vi "SO2 43i Serial Data Recording & DECADEv4.1.vi"() -> ()   [LabVIEW 2014]
uses:
  <vilib>/Instr/_visa.llb/VISA Set IO Buffer Mask.ctl
  <vilib>/Platform/TimedLoop/XDataNode/timing_clust.ctl
  <vilib>/Platform/TimedLoop/XDataNode/nitl_modes.ctl
  <vilib>/Platform/TimedLoop/XDataNode/wakeup.ctl
  C:/Program Files (x86)/National Instruments/LabVIEW 2014/examples/Data Communication/Network Streams/Simple Network Streams/support/Network Stream Command.ctl
  <vilib>/Utility/error.llb/whitespace.ctl
  <vilib>/Instr/_visa.llb/VISA Configure Serial Port (Instr).vi
  <vilib>/Utility/file.llb/Read From Spreadsheet File (string).vi
  <vilib>/Utility/tcp.llb/UDP Multicast Write-Only Open.vi
  <vilib>/platform/TimedLoop/XDataNode/XDataNode.xnode
  <vilib>/Platform/TimedLoop/XDataNode/XDNodeRunTimeDep.lvlib
  <vilib>/ptbypt/NI_PtbyPt.lvlib
panel:
  out "local\ndummy":bool
  out "cal gas cylinder conc":dbl=500.0 format="%.4g"
  out "calcon save to file":bool
  out "ev8 zero interval":i32=600
  out "Auto Zeroing":bool
  out "Simulate MOCCA Conc":dbl
  out "MOCCA window delay time (sec)":i32=30
  out "MOCCA SO2 Limit":i32=800
  out "SO2 Inflight MOCCA Alarm\n(default = OFF)":bool
  out "ev8 user set time":i32=60
  out "Mean Cal Offset":dbl
  out "Mean Cal\n(default = ON)":bool=TRUE
  out "Default file name":string
  out "Stop File Write":bool
  out "error out 4":errorcluster
  out "V6":bool
  out "V8":bool
  out "V9":bool
  out "error out 2":errorcluster
  in  "MFC_2 SLPM set value":dbl
  out "Value Read 2":string
  out "status 2":bool
  out "MFC 2":dbl[](array[numeric])
  in  "VISA resource name 3":refnum<visa-resource-name>="ASRL4::INSTR"
  in  "timeout (10sec) 3":u32=3000
  out "error out 3":errorcluster
  in  "MFC_3 SLPM set value":dbl=2.0
  out "Value Read 3":string
  out "status":bool
  out "MFC 3":dbl[](array[numeric])
  in  "VISA resource name 2":refnum<visa-resource-name>="ASRL5::INSTR"
  in  "timeout (10sec) 2":u32=3000
  out "Data Array UDP":string[](array[string])
  out "Slope":dbl=1.1
  out "Zero":dbl
  out "Simulate TWA Conc":dbl
  out "8hr_TWA_limit":i32=490
  out "10mins_STEL_limit":i32=800
  out "Simulate STEL Conc":dbl
  out "Simulate\nconc":bool
  out "q_size 2":i32
  out "8hr_so2_avg 2":dbl=1.0
  out "10min_so2_avg":dbl=1.0
  out "q_size":i32
  in  "Clear Display\nErrors":bool
  out "Data Processing":bool
  out "Serial Visa Error":errorcluster
  out "SEPTIC TCP Error Out":errorcluster
  out "TCP packet\nSend to SEPTIC":bool
  out "UDP Time Stamp Offset":i32=1
  out "Data Array TCP":string[](array[string])
  out "UDP packet \nstatus":bool
  out "UDP_Out_Error":errorcluster
  out "FISH TCP Error Out":errorcluster
  out "TCP packet\nSend to FISH":bool
  out "TCP Binary Packet":string
  out "Scan from String Error Counter\nfrom process loop":i32
  out "Read Error Counter\nfrom process loop":i32
  in  "milliseconds to wait":u32=330
  in  "ID":string="µ"
  in  "VISA resource name":refnum<visa-resource-name>="ASRL6::INSTR"
  out "Data In Array":string[](array[string])
  out "UDP_ASCII_Out":string
  out "UDP_Pack_num":u32
  out "Flight Number":string
  in  "dummy":string="00"
  out "Data String":string
  out "Internal packet":string[](array[string])
  out "RAW DATA":string
  in  "stop":bool
  out "Time taken history":u32(graph)
  out "Max Acq Time diff":u32
  out "Acq Time":u32
  out "Number of Send & Read Error\nfrom Acquire Loop":i32
  out "Command In":string
  # "SO2_conc"
  # "PMT_Volt"
  # "Lamp_Volt"
  # "Lamp_Intensity_Hz"
  # "Internal_Temp_degC"
  # "Reaction_Chamber_Temp_degC"
  # "Reaction_Chamber_Press_mmHg"
  # "Sample_Flow_litre_per_minute"
  # "Flag"
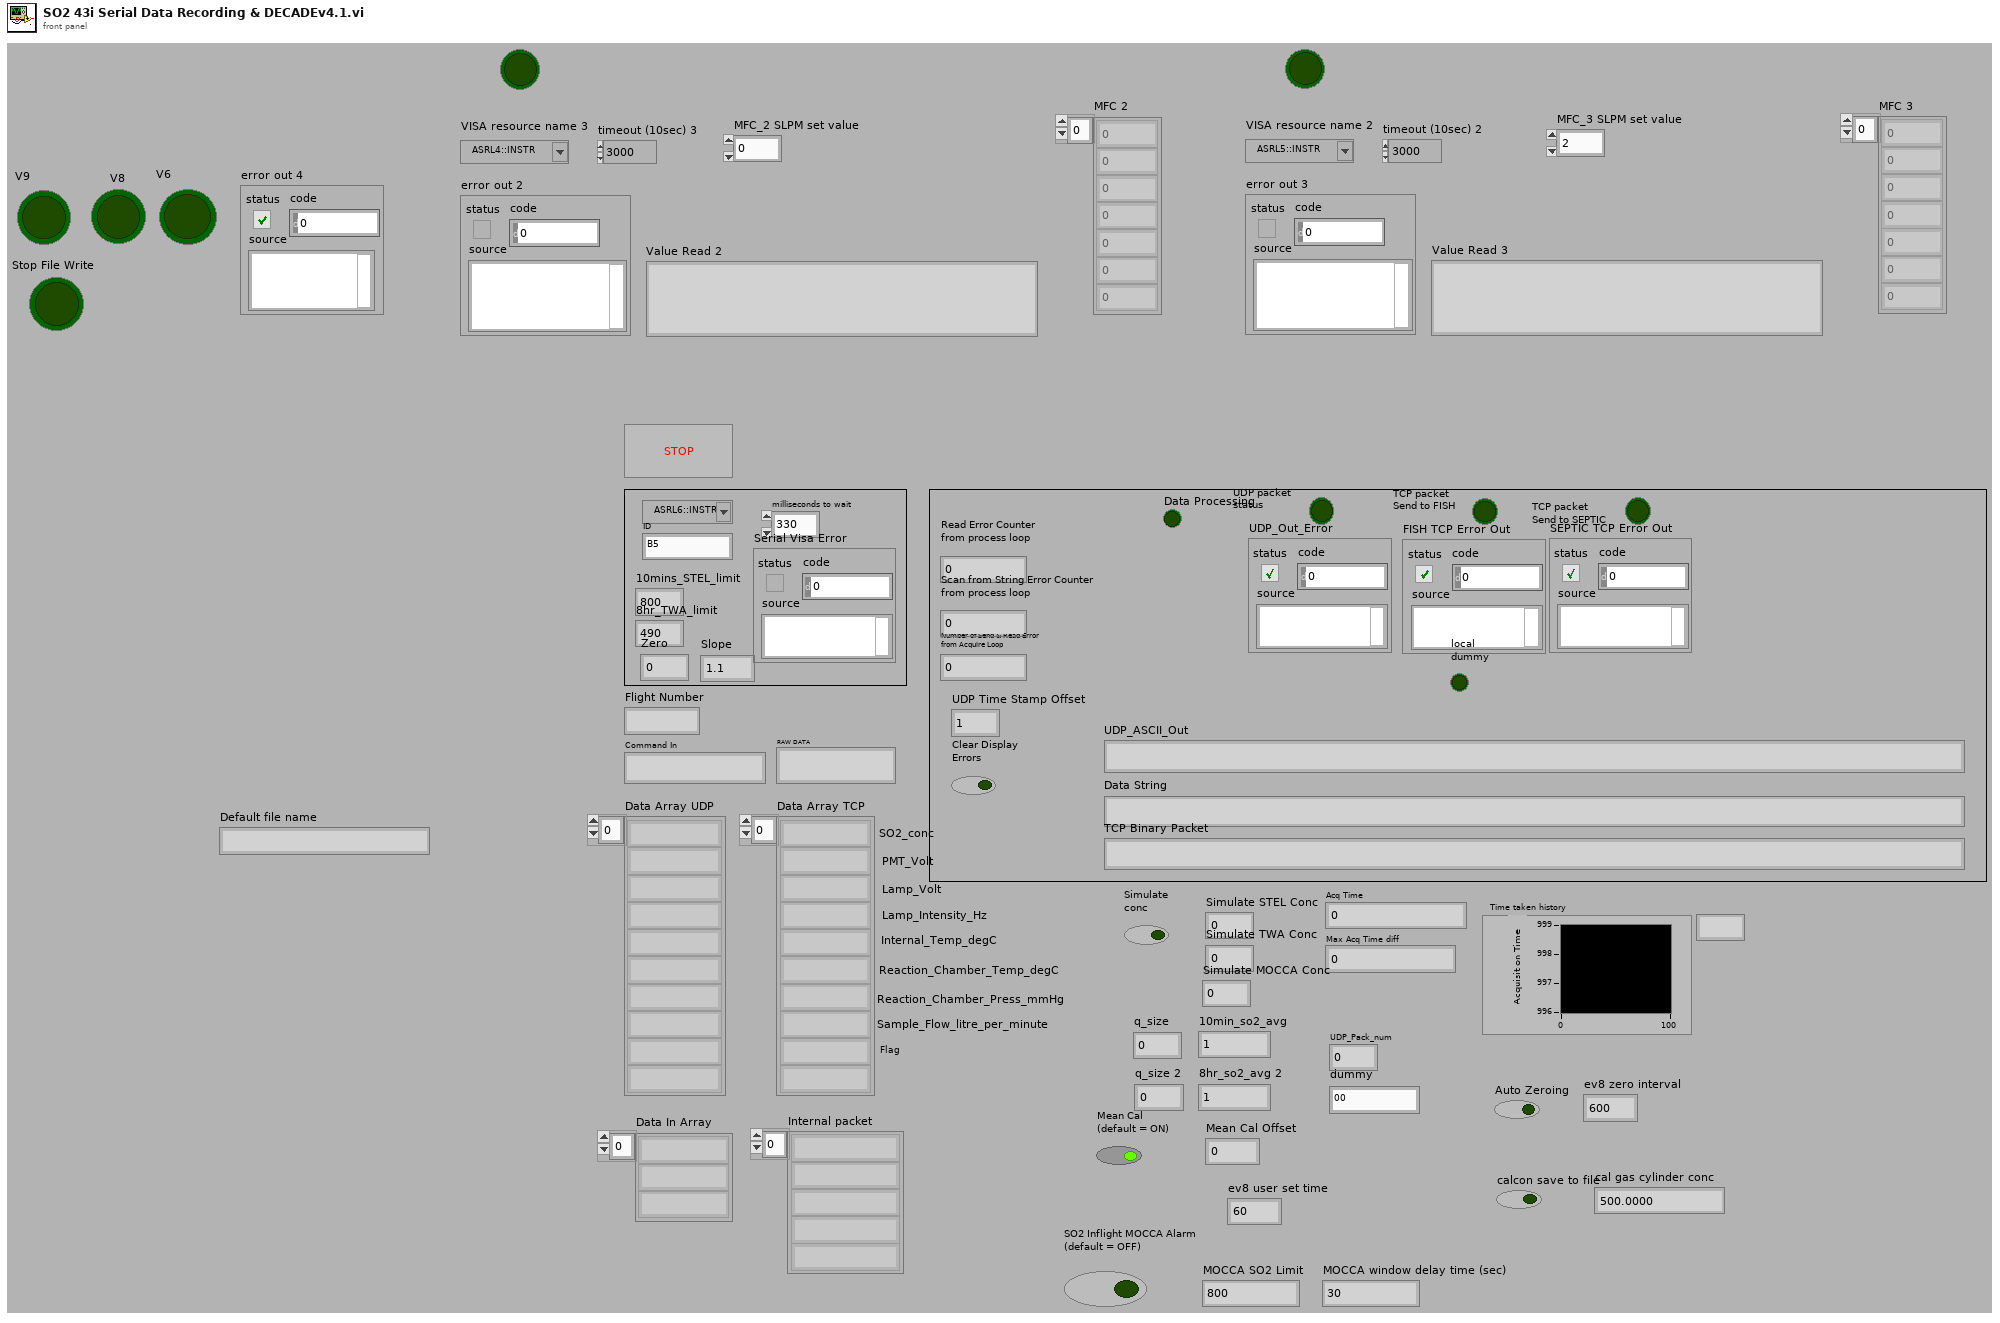
[diagram p1: front panel]
types:
  T1 = typedef "VISA Set IO Buffer Mask.ctl" = u16
  T2 = enum16{"open", "replace", "create", "open or create", "replace or create", "replace or create with confirmation"}
  T3 = typedef "Network Stream Command.ctl" = cluster{"Message":string, "Message Data":variant}
  T4 = typedef "XDNodeRunTimeDep.lvlib/timing_clust.ctl" = cluster{"Expected End [f-1]":u64, "Actual End [f-1]":u64, "Finished Late? [f-1]":bool, "Expected End [i-1]":u64, "Actual End [i-1]":u64, "Finished Late? [i-1]":bool, "Expected Start [i]":u64, "Actual Start [i]":u64, "Expected Start [f]":u64, "Actual Start [f]":u64, "Source Name":string, "Structure Name":string, "Period":i64, "Deadline":i64, "Offset":i64, "Start":i64, "Priority":i32, "Timeout":i32, "Mode":T5, "Wakeup Reason":T6, "Error":errorcluster, "Source Type":string, "Secondary Source Type":string, "Global End Time":u64, "Global Start Time":u64, "Frame Duration":u64, "Iteration Duration":u64, "Assigned CPU":i32, "I/O Scan Engine Mode":u32}
  T5 = typedef "XDNodeRunTimeDep.lvlib/nitl_modes.ctl" = enum32{"No Change", "Process missed periods, maintain original phase", "Discard missed periods, maintain original phase", "Process missed periods, ignore original phase", "Discard missed periods, ignore original phase"}
  T6 = typedef "XDNodeRunTimeDep.lvlib/wakeup.ctl" = enum32{"Normal", "Aborted", "Asynchronous wakeup", "Timing source error", "Timed loop error", "Timeout"}
  T7 = typedef "whitespace.ctl" = u16
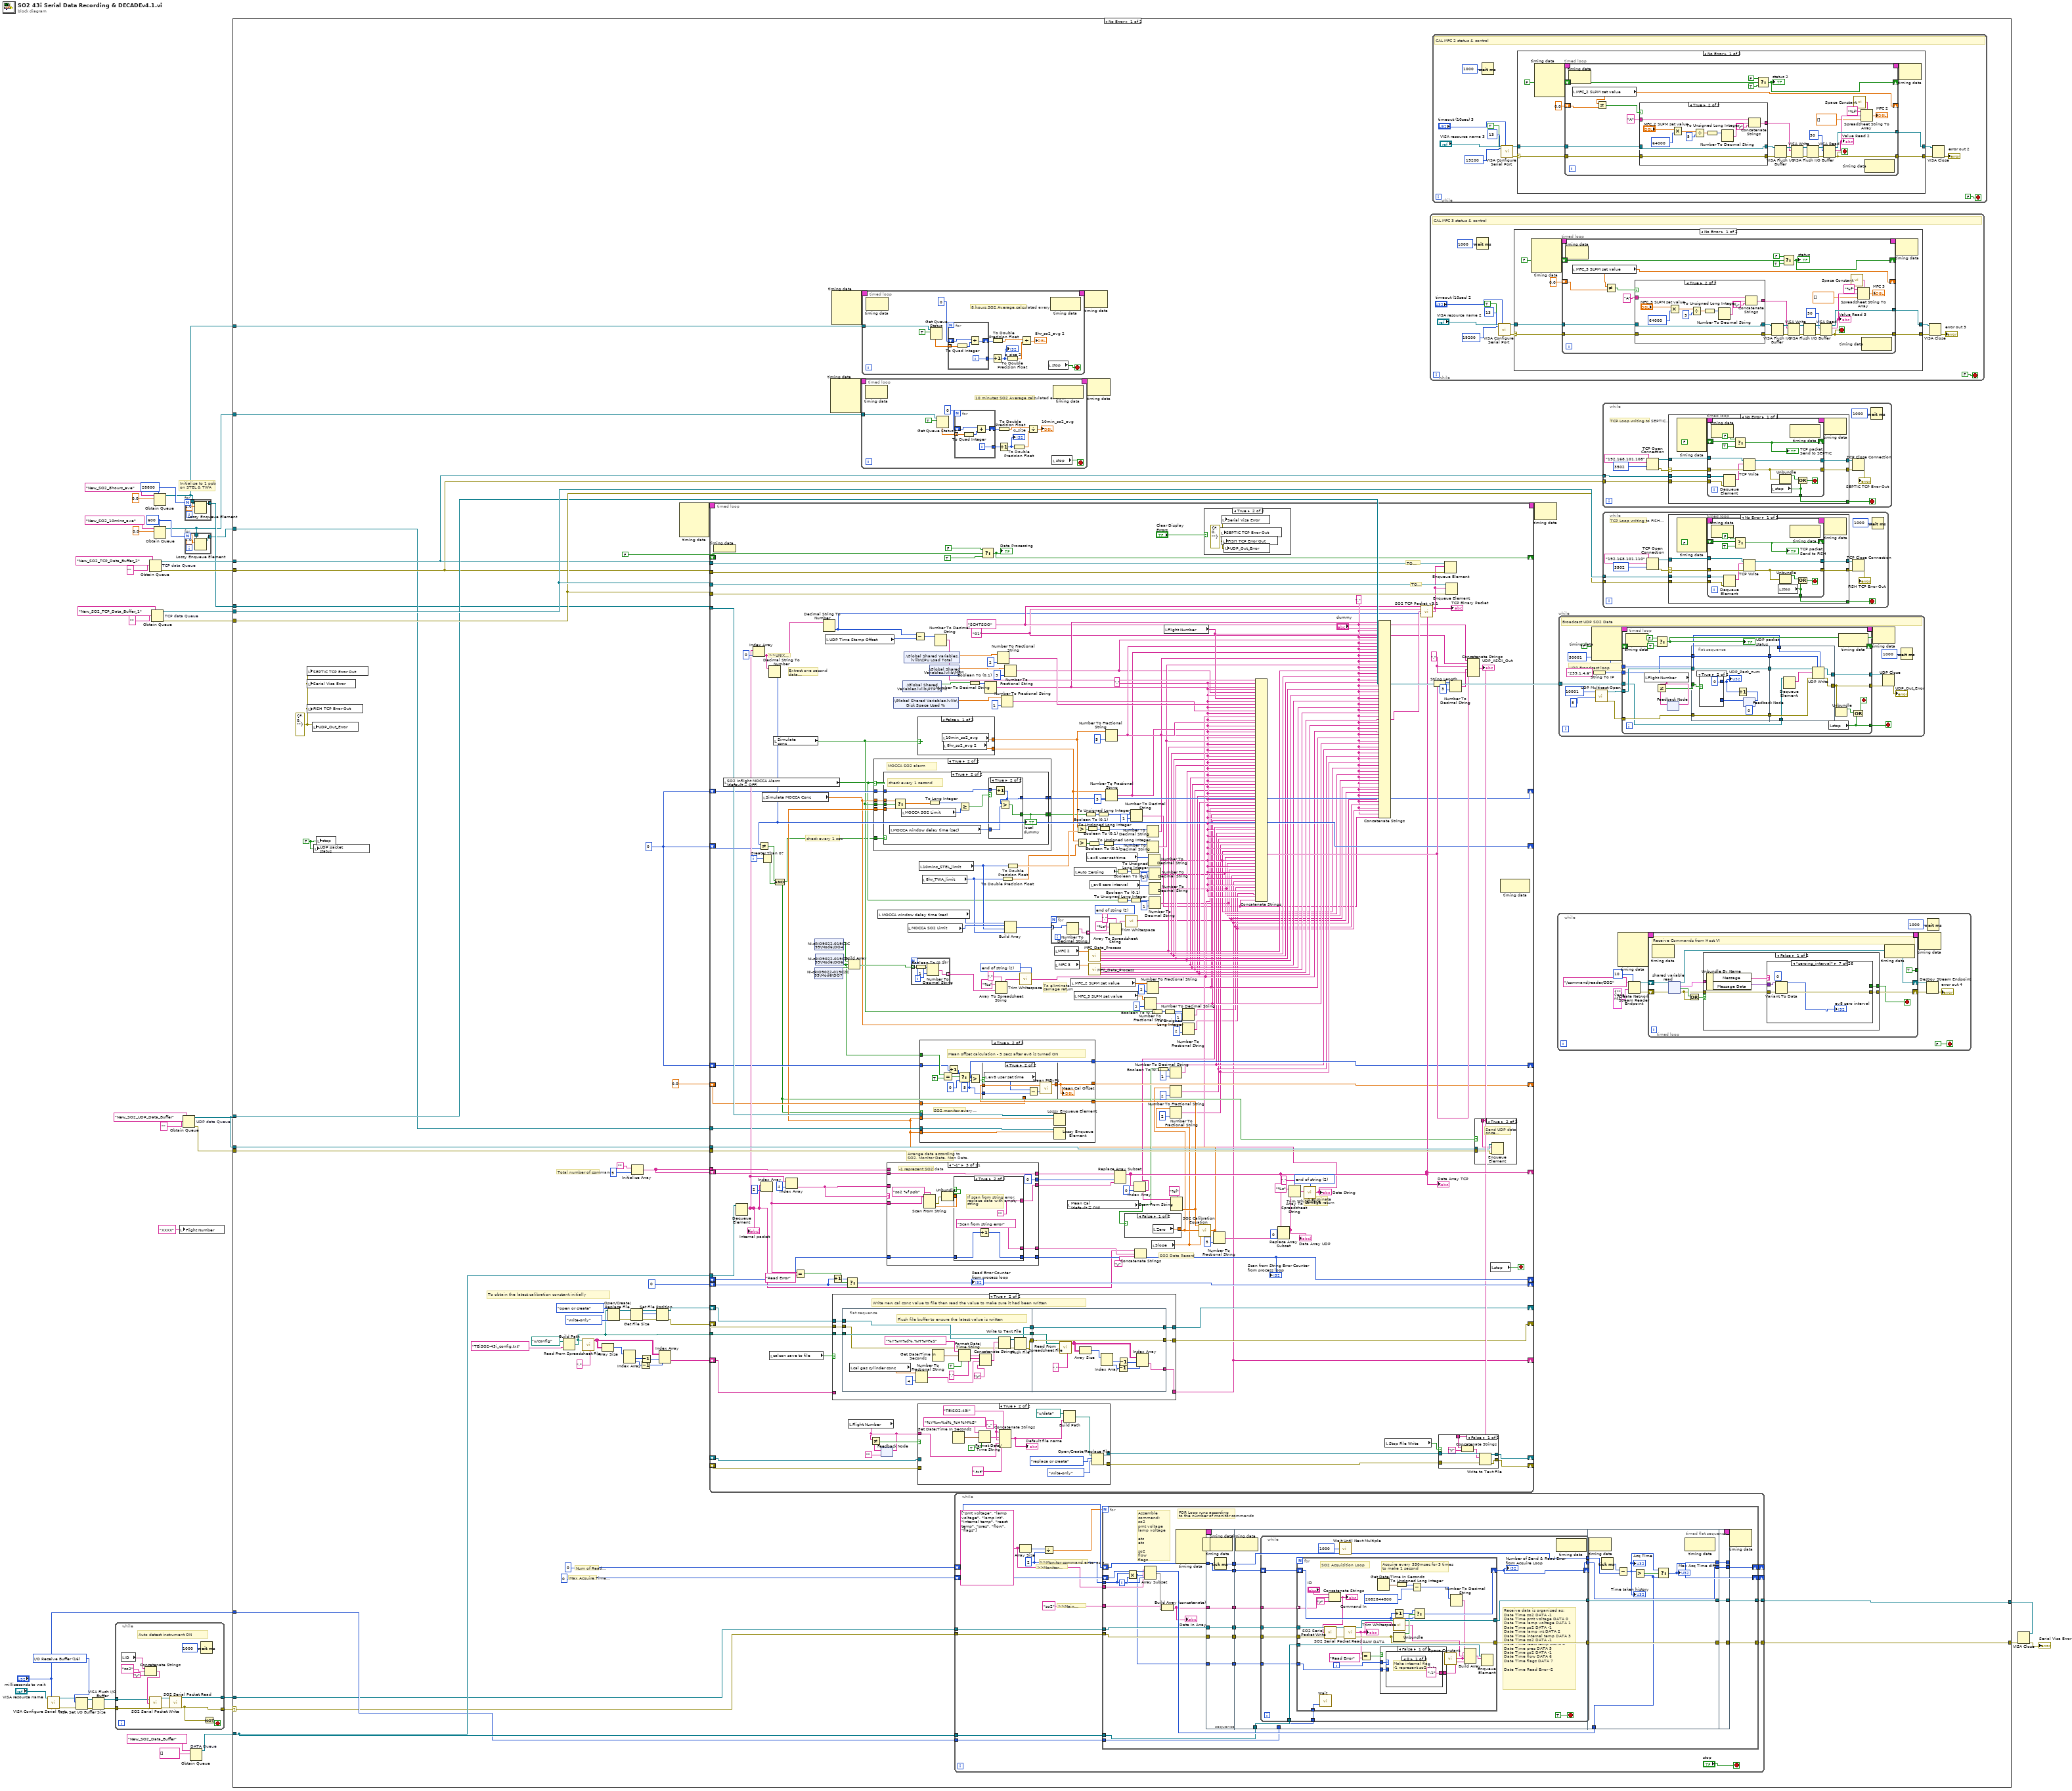
[diagram p0: block diagram]
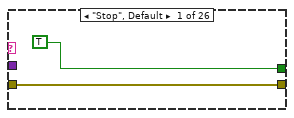
[diagram p2: hidden frame]
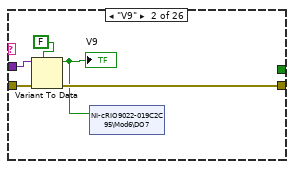
[diagram p3: hidden frame]
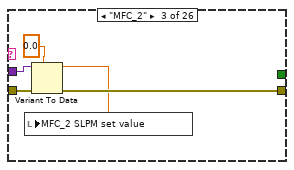
[diagram p4: hidden frame]
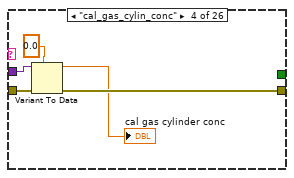
[diagram p5: hidden frame]
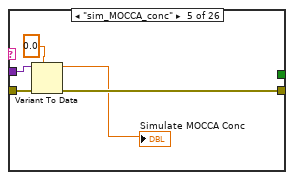
[diagram p6: hidden frame]
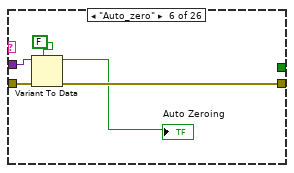
[diagram p7: hidden frame]
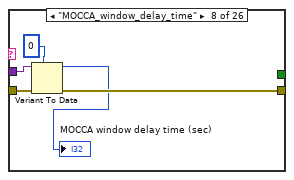
[diagram p8: hidden frame]
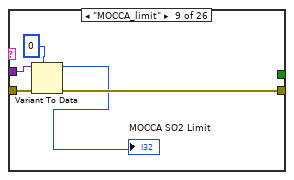
[diagram p9: hidden frame]
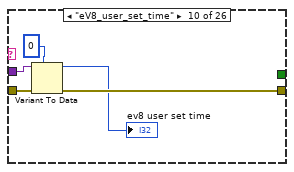
[diagram p10: hidden frame]
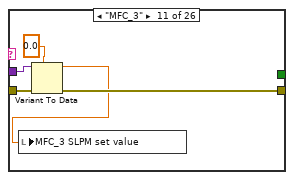
[diagram p11: hidden frame]
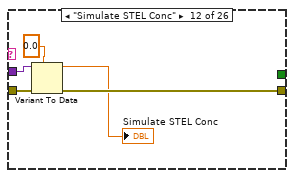
[diagram p12: hidden frame]
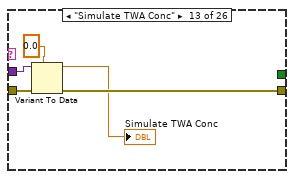
[diagram p13: hidden frame]
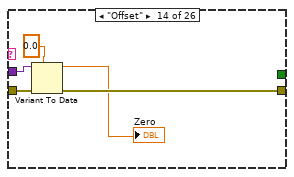
[diagram p14: hidden frame]
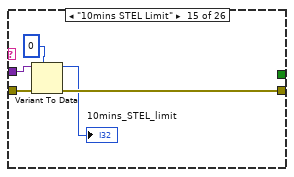
[diagram p15: hidden frame]
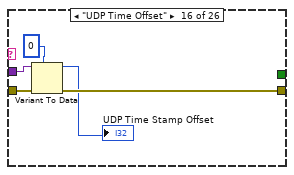
[diagram p16: hidden frame]
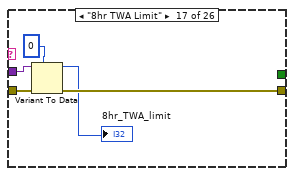
[diagram p17: hidden frame]
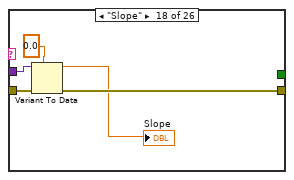
[diagram p18: hidden frame]
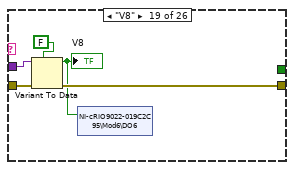
[diagram p19: hidden frame]
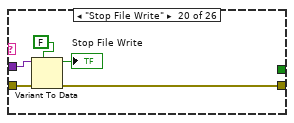
[diagram p20: hidden frame]
diagram:
  w9 = T1 16 items=["I/O Receive Buffer"=16, "I/O Transmit Buffer"=32, "I/O Receive and Transmit Buffer"=48] ("Mask")
  w16 = 28800 ("max queue size (-1, unlimited)")
  w13 = 600 ("max queue size (-1, unlimited)")
  # "Initialise to 1 ppb\non STEL & TWA"
  n1 = call-poly "VISA Configure Serial Port"("VISA resource name"="VISA resource name", "timeout (10sec)"="milliseconds to wait") -> ("VISA resource name out"=w8:refnum<visa-resource-name>, "error out"=w7:errorcluster)  [unwired: 12 in]
  n2 = VISA Set I/O Buffer Size(VISA resource name=w8, mask (16)=w9, error in (no error)=w7) -> (VISA resource name out=w2:refnum<visa-resource-name>, error out=w10:errorcluster)  [unwired: 1 in]
  n3 = VISA Flush I/O Buffer(VISA resource name=w2, error in (no error)=w10) -> (VISA resource name out=w6:refnum<visa-resource-name>, error out=w5:errorcluster)  [unwired: 1 in]
  n4 = while {
    tunnel: w6 -> [w45]
    tunnel: w5 -> [w44]
    tunnel: [w43] -> w4
    tunnel: [w42] -> w3
    stop <- w41 stop-if-true
    # "Auto detect instrument ON"
    n5 = local read "ID"() -> (w46:string)
    n6 = Concatenate Strings(w46, "so2" ("string"), "\r") -> (w49:string)
    n7 = call "SO2 Serial Packet Write.vi"("VISA resource name In"=w45, "Data in"=w49, "error in (no error)"=w44) -> ("VISA resource name Out"=w51:refnum<visa-resource-name>, "error out"=w50:errorcluster)  [unwired: 11 in]
    n8 = call "SO2 Serial Packet Read.vi"("VISA resource In"=w51, "error in"=w50) -> ("VISA resource Out"=w42:refnum<visa-resource-name>, "error out"=w43:errorcluster)  [unwired: 11 in, 1 out]
    n9 = Wait (ms)(milliseconds to wait=u32 1000) -> ()  [unwired: 1 out]
    n10 = Not(x=w43) -> (.not. x?=w41:bool)
  }
  n11 = Obtain Queue "TCP data Queue"(name (unnamed)="New_SO2_TCP_Data_Buffer_2", element data type="") -> (queue out=w23:refnum<queue>, error out=w22:errorcluster)  [unwired: 3 in, 1 out]
  n12 = Obtain Queue "TCP data Queue"(name (unnamed)="New_SO2_TCP_Data_Buffer_1", element data type="") -> (queue out=w31:refnum<queue>, error out=w30:errorcluster)  [unwired: 3 in, 1 out]
  n13 = Obtain Queue(max queue size (-1, unlimited)=w16, name (unnamed)="New_SO2_8hours_ave", element data type=0.0 ("index")) -> (queue out=w15:refnum<queue>)  [unwired: 2 in, 2 out]
  n14 = Obtain Queue(max queue size (-1, unlimited)=w13, name (unnamed)="New_SO2_10mins_ave", element data type=0.0 ("index")) -> (queue out=w12:refnum<queue>)  [unwired: 2 in, 2 out]
  n15 = local write "Flight Number"("XXXX" ("Flight Number")) -> ()
  n16 = Obtain Queue "UDP data Queue"(name (unnamed)="New_SO2_UDP_Data_Buffer", element data type="") -> (queue out=w26:refnum<queue>, error out=w27:errorcluster)  [unwired: 3 in, 1 out]
  n17 = for {
    N: w16 -> [_]
    tunnel: w15 -> [w55]
    tunnel: [w54] -> w14
    n18 = Lossy Enqueue Element(queue=w55, element=1.0) -> (queue out=w54:refnum<queue>)  [unwired: 1 in, 3 out]
  }
  n19 = for {
    N: w13 -> [_]
    tunnel: [w58] -> w11
    tunnel: w12 -> [w56]
    n20 = Lossy Enqueue Element(queue=w56, element=1.0) -> (queue out=w58:refnum<queue>)  [unwired: 1 in, 3 out]
  }
  n21 = Obtain Queue "DATA Queue"(name (unnamed)="New_SO2_Data_Buffer", element data type=string[] []) -> (queue out=w38:refnum<queue>)  [unwired: 3 in, 2 out]
  n22 = case shown="No Error" w4 {
    selector: w4 -> [w81 w1282]
    tunnel: [w112 w1282] -> w35
    tunnel: [w111 w1281] -> w36
    tunnel: w38 -> [w108 _]
    tunnel: w3 -> [w82 w1281]
    tunnel: w31 -> [w100 _]
    tunnel: w30 -> [w99 _]
    tunnel: w26 -> [w98 _]
    tunnel: w27 -> [w97 _]
    tunnel: w26 -> [w96 _]
    tunnel: w23 -> [w95 _]
    tunnel: w22 -> [w94 _]
    tunnel: "milliseconds to wait" -> [w93 _]
    tunnel: w12 -> [w90 _]
    tunnel: w15 -> [w89 _]
    tunnel: w11 -> [w88 _]
    tunnel: w14 -> [w87 _]
    frame No Error {
      w79 = 0
      w91 = errorcluster {"status"=FALSE, "code"=0, "source"=""} ("UDP Error Out")
      w102 = 0
      w101 = FALSE ("stop")
      # "To obtain the latest calibration constant initially"
      # "Max Acquire Time Diff"
      # "Num of Read Error"
      # "Total number of commands"
      n23 = local write "SEPTIC TCP Error Out"(w91) -> ()
      n24 = local write "Serial Visa Error"(w91) -> ()
      n25 = local write "FISH TCP Error Out"(w91) -> ()
      n26 = local write "UDP_Out_Error"(w91) -> ()
      n27 = local write "UDP packet \nstatus"(w101) -> ()
      n28 = local write "stop"(w101) -> ()
      n29 = Build Path(base path=path "u:/config", name or relative path="TEiSO2-43i_config.txt" ("string")) -> (appended path=w61:path)
      n30 = call-poly <vilib>:"Read From Spreadsheet File.vi"("delimiter (\\t)"="," ("delimiter (\\t)"), "file path (dialog if empty)"=w61) -> ("all rows"=w70:string[][])  [unwired: 5 in, 4 out]
      n31 = Array Size(array=w70) -> (size(s)=w71:i32[])
      n32 = Open/Create/Replace File(file path (use dialog)=w61, operation (0:open)=T2."open or create", access (0:read/write)=enum16{"read/write", "read-only", "write-only"}."write-only") -> (refnum out=w63:refnum<file>, error out=w64:errorcluster)  [unwired: 3 in, 1 out]
      n33 = Index Array(array=w71) -> (element #1=w75:i32, element #2=w73:i32)  [unwired: 2 in]
      n34 = Get File Size(file=w63, error in=w64) -> (refnum out=w65:refnum<file>, size (in bytes)=w67:i64, 0:w66:errorcluster)
      n35 = Initialize Array("", 9) -> (w103:string[])
      n36 = Decrement(x=w73) -> (x-1=w72:i32)
      n37 = Decrement(x=w75) -> (x-1=w74:i32)
      n38 = Set File Position(offset (in bytes) (0)=w67, refnum=w65, error in=w66) -> (refnum out=w60:refnum<file>, error out=w59:errorcluster)  [unwired: 1 in]
      n39 = Index Array(array=w70, index (row)=w74, index (col)=w72) -> (element=w69:string)
      n40 = node-c288() -> (w110:T4)  [unwired: 4 in]
      n41 = timed-loop {
        timing: w110 -> [_]
        timing-out: [_] -> w109
        tunnel: w108 -> [w940]
        shift-right: [w872] -> _
        shift-left: w103 -> [w930]
        shift-right: [w921] -> _
        shift-left: w102 -> [w918]
        tunnel: w103 -> [w920]
        shift-right: [w916] -> _
        shift-left: w102 -> [w917]
        tunnel: w100 -> [w914]
        tunnel: w99 -> [w913]
        tunnel: w98 -> [w912]
        tunnel: w97 -> [w911]
        shift-right: [w903] -> _
        shift-left: w79 -> [w906]
        tunnel: w95 -> [w902]
        tunnel: w94 -> [w901]
        shift-right: [w894] -> _
        shift-left: FALSE -> [w897]
        tunnel: w88 -> [w891]
        tunnel: w87 -> [w890]
        shift-right: [w859] -> _
        shift-left: _ -> [w861]
        shift-right: [w858] -> _
        shift-left: _ -> [w860]
        shift-right: [w828] -> _
        shift-left: w79 -> [w830]
        shift-right: [w826] -> _
        shift-left: 0.0 -> [w827]
        shift-right: [w816] -> _
        shift-left: w79 -> [w817]
        tunnel: w61 -> [w793]
        shift-right: [w747] -> _
        shift-left: w69 -> [w792]
        shift-right: [w783] -> _
        shift-left: w60 -> [w784]
        shift-right: [w781] -> _
        shift-left: w59 -> [w782]
        i -> [w904]
        stop <- w938 stop-if-true
        w744 = ","
        (unwired) i16 1 ("width (-)")
        (unwired) T7 2 items=["both", "start of string", "end of string"] ("location (both)")
        w836 = T7 2 items=["both", "start of string", "end of string"] ("location (both)")
        w926 = T7 2 items=["both", "start of string", "end of string"] ("location (both)")
        w786 = ","
        w740 = "01"
        w932 = ","
        w741 = "$CHTSOO"
        # "check every 1 sec"
        # "To eliminate\ncarriage return"
        # "TO SEPTIC"
        # "TO FISH"
        # "Extract one second data\nfor UDP sending"
        # "Arrange data according to\nSO2, Monitor Data, Mon Data,"
        # "To eliminate\ncarriage return"
        # ">>UNIX TIME>>"
        # "SO2 Data Record"
        n42 = node-c288() -> ()  [unwired: 1 in]
        n43 = local read "SO2 Inflight MOCCA Alarm\n(default = OFF)"() -> (w779:bool)
        n44 = Dequeue Element(queue=w940) -> (element=w909:string[])  [unwired: 2 in, 3 out]
        "Internal packet" <- w909
        n45 = Index Array(array=w909, index=0) -> (element=w908:string)
        n46 = Index Array(array=w909, index=2) -> (element=w924:string)
        n47 = Greater Than 0?(x=w904) -> (x > 0?=w907:bool)
        n48 = local read "Simulate MOCCA Conc"() -> (w787:dbl)
        n49 = Decimal String To Number(string=w908) -> (number=w903:i32)  [unwired: 2 in, 1 out]
        n50 = Not Equal?(x=w903, y=w906) -> (x != y?=w905:bool)
        n51 = local read "calcon save to file"() -> (w780:bool)
        n52 = local read "Simulate\nconc"() -> (w789:bool)
        n53 = Compound Arithmetic op=AND(w905, w907) -> (w778:bool)
        n54 = Index Array(array=w909, index=4) -> (element=w893:string)
        n55 = Equal?(x=w924, y="Read Error") -> (x = y?=w922:bool)
        n56 = shared-variable "NI-cRIO9022-019C2C95\\Mod6\\DO7"() -> (w844:bool)  [unwired: 1 in, 1 out]
        n57 = shared-variable "NI-cRIO9022-019C2C95\\Mod6\\DO4"() -> (w845:bool)  [unwired: 1 in, 1 out]
        n58 = shared-variable "NI-cRIO9022-019C2C95\\Mod6\\DO6"() -> (w831:bool)  [unwired: 1 in, 1 out]
        n59 = Decimal String To Number(string=w908) -> (number=w739:i32)  [unwired: 2 in, 1 out]
        n60 = local read "UDP Time Stamp Offset"() -> (w835:i32)
        n61 = Increment(x=w918) -> (x+1=w919:i32)
        n62 = case shown="True" w780 {
          tunnel: w793 -> [_ w952]
          tunnel: [w941 w950] -> w781
          tunnel: w792 -> [w943 _]
          tunnel: [w943 w949] -> w747
          tunnel: w784 -> [w942 w947]
          tunnel: [w942 w945] -> w783
          tunnel: w782 -> [w941 w944]
          frame False {
          }
          frame True {
            # "Write new cal conc value to file then read the value to make sure it had been written"
            n63 = flat-sequence {
              tunnel: w952 -> [w960]
              tunnel: [w955] -> w951
              tunnel: [w960] -> w948
              tunnel: w947 -> [w959]
              tunnel: [w954] -> w946
              tunnel: w944 -> [w958]
              tunnel: w951 -> [w973]
              tunnel: [w973] -> w950
              tunnel: [w972] -> w949
              tunnel: w948 -> [w971]
              tunnel: w946 -> [w970]
              tunnel: [w970] -> w945
              frame #0 {
                # "Flush file buffer to ensure the latest value is written"
                n64 = local read "cal gas cylinder conc"() -> (w953:dbl)
                n65 = Number To Fractional String(number=w953, precision (6)=i16 4) -> (F-format string=w961:string)  [unwired: 2 in]
                n66 = Get Date/Time In Seconds() -> (seconds since 1Jan1904=w968:timestamp)
                n67 = Format Date/Time String(time format string (%c)="%Y%m%d%,%H%M%S", seconds (now)=w968, UTC format=TRUE) -> (date/time string=w965:string)
                n68 = Concatenate Strings(w965, "," ("string"), w961, "\r") -> (w963:string)
                n69 = Write to Text File(file (use dialog)=w959, text=w963, error in=w958) -> (refnum out=w956:refnum<file>, error out=w957:errorcluster)  [unwired: 1 in, 1 out]
                n70 = Flush File(refnum=w956, error in=w957) -> (refnum out=w954:refnum<file>, error out=w955:errorcluster)
              }
              frame #1 {
                n71 = call-poly <vilib>:"Read From Spreadsheet File.vi"("delimiter (\\t)"="," ("delimiter (\\t)"), "file path (dialog if empty)"=w971) -> ("all rows"=w974:string[][])  [unwired: 5 in, 4 out]
                n72 = Array Size(array=w974) -> (size(s)=w975:i32[])
                n73 = Index Array(array=w975) -> (element #1=w979:i32, element #2=w977:i32)  [unwired: 2 in]
                n74 = Decrement(x=w977) -> (x-1=w976:i32)
                n75 = Decrement(x=w979) -> (x-1=w978:i32)
                n76 = Index Array(array=w974, index (row)=w978, index (col)=w976) -> (element=w972:string)
              }
            }
          }
        }
        n77 = Select(t=w919, s=w922, f=w918) -> (s? t:f=w921:i32)
        "Read Error Counter\nfrom process loop" <- w921
        n78 = Build Array(w845, w831, w844) -> (w849:bool[])
        n79 = local read "Flight Number"() -> (w862:string)
        n80 = local read "MOCCA window delay time (sec)"() -> (w798:i32)
        n81 = feedback #1("" ("Flight Number")) -> (w867:string)
        n82 = Not Equal?(x=w862, y=w867) -> (x != y?=w865:bool)
        n83 = feedback-in #1(w862) -> ()
        n84 = case shown="\"-1\"" w893 {
          tunnel: w893 -> [w1080 _ _ w1116 w1137 w1158 w1180 w1202 w1224 w1246 w1268]
          tunnel: w930 -> [w1081 _ w1095 w1117 w1138 w1159 w1181 w1203 w1225 w1247 w1269]
          tunnel: w924 -> [_ _ w1092 w1112 w1133 w1155 w1177 w1199 w1221 w1243 w1265]
          tunnel: [w1081 w1084 w1095 w1117 w1138 w1159 w1181 w1203 w1225 w1247 w1269] -> w877
          tunnel: [w1078 _ 0 ("index") w1114 w1135 w1156 w1178 w1200 w1222 w1244 w1266] -> w876
          tunnel: [_ _ w1091 w1111 w1132 w1154 w1176 w1198 w1220 w1242 w1260] -> w929
          tunnel: w920 -> [_ w1084 _ _ _ _ _ _ _ _ _]
          tunnel: w917 -> [w1076 w1083 w1088 w1108 w1129 w1149 w1172 w1193 w1216 w1237 w1259]
          tunnel: [w1076 w1083 w1087 w1107 w1128 w1148 w1171 w1192 w1215 w1236 w1258] -> w916
          tunnel: ["Internal False Flag Detected" "" w1086 w1106 w1127 w1147 w1170 w1191 w1214 w1235 w1257] -> w915
          frame "False", Default {
            n85 = Decimal String To Number(string=w1080) -> (number=w1077:i32)  [unwired: 2 in, 1 out]
            n86 = Add(x=w1077, y=1) -> (x+y=w1078:i32)
          }
          frame "-2" {
            # "Read Error Detected\nMake all data as a space"
          }
          frame "-1" {
            # "-1 represent SO2 data"
            n87 = Scan From String(format string="so2 %f ppb", input string=w1092) -> (error out=w1090:errorcluster, output 1=w1085:dbl)  [unwired: 3 in, 2 out]
            n88 = Unbundle(w1090) -> ("status"=w1089:bool)  [unwired: 2 out]
            n89 = case shown="True" w1089 {
              tunnel: w1085 -> [w1096 _]
              tunnel: [w1100 ""] -> w1091
              tunnel: w1088 -> [w1099 w1104]
              tunnel: [w1099 w1103] -> w1087
              tunnel: ["" "Scan from string error"] -> w1086
              frame False {
                # "Extract the concentration\nvalue & fixed format"
                n90 = Number To Fractional String(number=w1096, precision (6)=i16 5) -> (F-format string=w1100:string)  [unwired: 2 in]
              }
              frame True {
                # "If scan from string error,\nreplace data with empty\nstring"
                n91 = Increment(x=w1104) -> (x+1=w1103:i32)
              }
            }
          }
          frame "0" {
            # "0 represents pmt voltage -0510 volts"
            n92 = Scan From String(format string="pmt voltage %d", input string=w1112) -> (error out=w1110:errorcluster, output 1=w1105:i32)  [unwired: 3 in, 2 out]
            n93 = Decimal String To Number(string=w1116) -> (number=w1115:i32)  [unwired: 2 in, 1 out]
            n94 = Unbundle(w1110) -> ("status"=w1109:bool)  [unwired: 2 out]
            n95 = case shown="False" w1109 {
              tunnel: w1105 -> [w1121 _]
              tunnel: [w1118 w1122] -> w1111
              tunnel: w1108 -> [w1120 w1125]
              tunnel: [w1120 w1124] -> w1107
              tunnel: ["" "Scan from string error"] -> w1106
              tunnel: [w1118 w1122] -> _
              frame False {
                # "Extract the actual value\n& fixed format"
                n96 = Number To Decimal String(number=w1121) -> (decimal integer string=w1118:string)  [unwired: 1 in]
              }
              frame True {
                w1122 = ""
                # "If scan from string error,\nreplace data with empty\nstring"
                n97 = Increment(x=w1125) -> (x+1=w1124:i32)
              }
            }
            n98 = Increment(x=w1115) -> (x+1=w1114:i32)
          }
          frame "1" {
            # "1 represents lamp voltage; lamp voltage 810 volts"
            n99 = Scan From String(format string="lamp voltage %d", input string=w1133) -> (error out=w1131:errorcluster, output 1=w1126:i32)  [unwired: 3 in, 2 out]
            n100 = Decimal String To Number(string=w1137) -> (number=w1136:i32)  [unwired: 2 in, 1 out]
            n101 = Unbundle(w1131) -> ("status"=w1130:bool)  [unwired: 2 out]
            n102 = case shown="True" w1130 {
              tunnel: w1126 -> [w1142 _]
              tunnel: [w1139 w1143] -> w1132
              tunnel: w1129 -> [w1141 w1146]
              tunnel: [w1141 w1145] -> w1128
              tunnel: ["" "Scan from string error"] -> w1127
              tunnel: [w1139 w1143] -> _
              frame False {
                # "Extract the actual value\n& fixed format"
                n103 = Number To Decimal String(number=w1142) -> (decimal integer string=w1139:string)  [unwired: 1 in]
              }
              frame True {
                w1143 = ""
                # "If scan from string error,\nreplace data with empty\nstring"
                n104 = Increment(x=w1146) -> (x+1=w1145:i32)
              }
            }
            n105 = Increment(x=w1136) -> (x+1=w1135:i32)
          }
          frame "2" {
            # "2 represents lamp intensity; lamp int 35867 Hz"
            n106 = Scan From String(format string="lamp int %d", input string=w1155) -> (error out=w1151:errorcluster, output 1=w1152:i32)  [unwired: 3 in, 2 out]
            n107 = Decimal String To Number(string=w1158) -> (number=w1157:i32)  [unwired: 2 in, 1 out]
            n108 = Unbundle(w1151) -> ("status"=w1150:bool)  [unwired: 2 out]
            n109 = case shown="True" w1150 {
              tunnel: [w1160 w1165] -> w1154
              tunnel: w1152 -> [w1164 _]
              tunnel: w1149 -> [w1163 w1168]
              tunnel: [w1163 w1167] -> w1148
              tunnel: ["" "Scan from string error"] -> w1147
              tunnel: [w1160 w1165] -> _
              frame False {
                # "Extract the actual value\n& fixed format"
                n110 = Number To Fractional String(number=w1164, precision (6)=i16 0) -> (F-format string=w1160:string)  [unwired: 2 in]
              }
              frame True {
                w1165 = ""
                # "If scan from string error,\nreplace data with empty\nstring"
                n111 = Increment(x=w1168) -> (x+1=w1167:i32)
              }
            }
            n112 = Increment(x=w1157) -> (x+1=w1156:i32)
          }
          frame "3" {
            # "3 represents internal temp; internal temp 027.2 deg C, actual 027.2"
            n113 = Scan From String(format string="%[^,], %s %f", input string=w1177) -> (error out=w1174:errorcluster, output 3=w1169:dbl)  [unwired: 7 in, 2 out]
            n114 = Decimal String To Number(string=w1180) -> (number=w1179:i32)  [unwired: 2 in, 1 out]
            n115 = Unbundle(w1174) -> ("status"=w1173:bool)  [unwired: 2 out]
            n116 = case shown="True" w1173 {
              tunnel: [w1182 w1187] -> w1176
              tunnel: w1169 -> [w1186 _]
              tunnel: w1172 -> [w1185 w1190]
              tunnel: [w1185 w1189] -> w1171
              tunnel: ["" "Scan from string error"] -> w1170
              tunnel: [w1182 w1187] -> _
              frame False {
                # "Extract the actual value\n& fixed format"
                n117 = Number To Fractional String(number=w1186, precision (6)=i16 1) -> (F-format string=w1182:string)  [unwired: 2 in]
              }
              frame True {
                w1187 = ""
                # "If scan from string error,\nreplace data with empty\nstring"
                n118 = Increment(x=w1190) -> (x+1=w1189:i32)
              }
            }
            n119 = Increment(x=w1179) -> (x+1=w1178:i32)
          }
          frame "4" {
            # "4 represents react temp; react temp 045.2 deg C"
            n120 = Scan From String(format string="react temp %f deg C", input string=w1199) -> (error out=w1195:errorcluster, output 1=w1196:dbl)  [unwired: 3 in, 2 out]
            n121 = Decimal String To Number(string=w1202) -> (number=w1201:i32)  [unwired: 2 in, 1 out]
            n122 = Unbundle(w1195) -> ("status"=w1194:bool)  [unwired: 2 out]
            n123 = case shown="False" w1194 {
              tunnel: [w1204 w1209] -> w1198
              tunnel: w1196 -> [w1208 _]
              tunnel: w1193 -> [w1207 w1212]
              tunnel: [w1207 w1211] -> w1192
              tunnel: ["" "Scan from string error"] -> w1191
              tunnel: [w1204 w1209] -> _
              frame False {
                # "Extract the actual value\n& fixed format"
                n124 = Number To Fractional String(number=w1208, precision (6)=i16 1) -> (F-format string=w1204:string)  [unwired: 2 in]
              }
              frame True {
                w1209 = ""
                # "If scan from string error,\nreplace data with empty\nstring"
                n125 = Increment(x=w1212) -> (x+1=w1211:i32)
              }
            }
            n126 = Increment(x=w1201) -> (x+1=w1200:i32)
          }
          frame "5" {
            # "5 represents chamber pressure; pres 760.0 mm Hg, actual 753.4"
            n127 = Scan From String(format string="%[^,], %s %f", input string=w1221) -> (error out=w1218:errorcluster, output 3=w1213:dbl)  [unwired: 7 in, 2 out]
            n128 = Decimal String To Number(string=w1224) -> (number=w1223:i32)  [unwired: 2 in, 1 out]
            n129 = Unbundle(w1218) -> ("status"=w1217:bool)  [unwired: 2 out]
            n130 = case shown="False" w1217 {
              tunnel: [w1226 w1231] -> w1220
              tunnel: w1213 -> [w1230 _]
              tunnel: w1216 -> [w1229 w1234]
              tunnel: [w1229 w1233] -> w1215
              tunnel: ["" "Scan from string error"] -> w1214
              tunnel: [w1226 w1231] -> _
              frame False {
                # "Extract the actual value\n& fixed format"
                n131 = Number To Fractional String(number=w1230, precision (6)=i16 1) -> (F-format string=w1226:string)  [unwired: 2 in]
              }
              frame True {
                w1231 = ""
                # "If scan from string error,\nreplace data with empty\nstring"
                n132 = Increment(x=w1234) -> (x+1=w1233:i32)
              }
            }
            n133 = Increment(x=w1223) -> (x+1=w1222:i32)
          }
          frame "6" {
            # "6 represents flow data; flow 0.503 l/m"
            n134 = Scan From String(format string="flow %f l/m", input string=w1243) -> (error out=w1239:errorcluster, output 1=w1240:dbl)  [unwired: 3 in, 2 out]
            n135 = Decimal String To Number(string=w1246) -> (number=w1245:i32)  [unwired: 2 in, 1 out]
            n136 = Unbundle(w1239) -> ("status"=w1238:bool)  [unwired: 2 out]
            n137 = case shown="True" w1238 {
              tunnel: [w1252 ""] -> w1242
              tunnel: w1240 -> [w1251 _]
              tunnel: w1237 -> [w1250 w1255]
              tunnel: [w1250 w1254] -> w1236
              tunnel: ["" "Scan from string error"] -> w1235
              frame False {
                # "Extract the actual value\n& fixed format"
                n138 = Number To Fractional String(number=w1251, precision (6)=i16 3) -> (F-format string=w1252:string)  [unwired: 2 in]
              }
              frame True {
                # "If scan from string error,\nreplace data with empty\nstring"
                n139 = Increment(x=w1255) -> (x+1=w1254:i32)
              }
            }
            n140 = Increment(x=w1245) -> (x+1=w1244:i32)
          }
          frame "7" {
            # "7 represents flags data; flags 1c100000"
            n141 = Scan From String(format string="flags %s", input string=w1265) -> (error out=w1263:errorcluster, output 1=w1261:string)  [unwired: 3 in, 2 out]
            n142 = Decimal String To Number(string=w1268) -> (number=w1267:i32)  [unwired: 2 in, 1 out]
            n143 = Unbundle(w1263) -> ("status"=w1262:bool)  [unwired: 2 out]
            n144 = case shown="False" w1262 {
              tunnel: w1261 -> [w1272 _]
              tunnel: [w1272 ""] -> w1260
              tunnel: w1259 -> [w1271 w1275]
              tunnel: [w1271 w1274] -> w1258
              tunnel: ["" "Scan from string error"] -> w1257
              frame False {
                # "Extract the actual value\n& fixed format"
              }
              frame True {
                # "If scan from string error,\nreplace data with empty\nstring"
                n145 = Increment(x=w1275) -> (x+1=w1274:i32)
              }
            }
            n146 = Increment(x=w1267) -> (x+1=w1266:i32)
          }
        }
        "Scan from String Error Counter\nfrom process loop" <- w916
        n147 = shared-variable ".\\Global Shared Variables.lvlib\\Disk Space Used %"() -> (w838:dbl)  [unwired: 1 in, 1 out]
        n148 = shared-variable ".\\Global Shared Variables.lvlib\\PTP Sync"() -> (w851:bool)  [unwired: 1 in, 1 out]
        n149 = shared-variable ".\\Global Shared Variables.lvlib\\CPU Load Total"() -> (w855:dbl)  [unwired: 1 in, 1 out]
        n150 = local read "MOCCA SO2 Limit"() -> (w797:i32)
        n151 = for {
          tunnel: w849 -> [w1019] mode=indexing
          tunnel: [w1018] -> w846 mode=indexing
          n152 = Boolean To (0,1)(Boolean=w1019) -> (0, 1=w1020:i16)
          n153 = Number To Decimal String(number=w1020, width (-)=i16 1) -> (decimal integer string=w1018:string)
        }
        n154 = Subtract(x=w739, y=w835) -> (x-y=w899:i32)
        n155 = case shown="False" w789 {
          tunnel: [w1012 w1013] -> w886
          tunnel: [w1011 w1014] -> w884
          frame False {
            n156 = local read "10min_so2_avg"() -> (w1012:dbl)
            n157 = local read "8hr_so2_avg 2"() -> (w1011:dbl)
          }
          frame True {
            # "SO2 STEL & TWA simulate"
            n158 = local read "Simulate STEL Conc"() -> (w1013:dbl)
            n159 = local read "Simulate TWA Conc"() -> (w1014:dbl)
          }
        }
        n160 = case shown="True" w865 {
          tunnel: [w1022 w1025] -> w864
          tunnel: [w1021 w1024] -> w863
          tunnel: w861 -> [w1022 _]
          tunnel: w860 -> [w1021 _]
          tunnel: w862 -> [_ w1023]
          frame False {
          }
          frame True {
            w1032 = "_" ("string")
            n161 = Get Date/Time In Seconds() -> (seconds since 1Jan1904=w1033:timestamp)
            n162 = Format Date/Time String(time format string (%c)="%Y%m%d%_%H%M%S", seconds (now)=w1033, UTC format=TRUE) -> (date/time string=w1036:string)
            n163 = Concatenate Strings("TEiSO2-43i" ("string"), w1032, w1036, w1032, w1023, ".txt" ("string")) -> (w1030:string)
            "Default file name" <- w1030
            n164 = Build Path(base path=path "u:/data", name or relative path=w1030) -> (appended path=w1026:path)
            n165 = Open/Create/Replace File(file path (use dialog)=w1026, operation (0:open)=T2."replace or create", access (0:read/write)=enum16{"read/write", "read-only", "write-only"}."write-only") -> (refnum out=w1025:refnum<file>, error out=w1024:errorcluster)  [unwired: 3 in, 1 out]
          }
        }
        n166 = local read "10mins_STEL_limit"() -> (w796:i32)
        n167 = local read "8hr_TWA_limit"() -> (w795:i32)
        n168 = shared-variable ".\\Global Shared Variables.lvlib\\MFM"() -> (w852:dbl)  [unwired: 1 in, 1 out]
        n169 = Number To Decimal String(number=w899) -> (decimal integer string=w898:string)  [unwired: 1 in]
        n170 = Boolean To (0,1)(Boolean=w851) -> (0, 1=w850:i16)
        n171 = Select(t=FALSE, s=w897, f=TRUE) -> (s? t:f=w894:bool)
        "Data Processing" <- w894
        n172 = Number To Decimal String(number=w850) -> (decimal integer string=w777:string)  [unwired: 1 in]
        n173 = Array To Spreadsheet String(delimiter (Tab)=",", array=w846, 3:"%s" ("format string")) -> (spreadsheet string=w837:string)
        n174 = Number To Fractional String(number=w855, precision (6)=i16 2) -> (F-format string=w834:string)  [unwired: 2 in]
        n175 = Number To Fractional String(number=w838, precision (6)=i16 1) -> (F-format string=w833:string)  [unwired: 2 in]
        n176 = To Double Precision Float(number=w795) -> (double precision float=w887:dbl)
        n177 = Number To Fractional String(number=w852, precision (6)=i16 3) -> (F-format string=w769:string)  [unwired: 2 in]
        n178 = Build Array(w798, w797, w796, w795) -> (w794:i32[])
        n179 = To Double Precision Float(number=w796) -> (double precision float=w888:dbl)
        n180 = call <vilib>:"Trim Whitespace.vi"("string"=w837, "location (both)"=w836) -> ("trimmed string"=w758:string)
        n181 = for {
          tunnel: w794 -> [w981] mode=indexing
          tunnel: [w982] -> w800 mode=indexing
          n182 = Number To Decimal String(number=w981) -> (decimal integer string=w982:string)  [unwired: 1 in]
        }
        n183 = local read "MFC 2"() -> (w869:dbl[])
        n184 = local read "MFC 3"() -> (w868:dbl[])
        n185 = local read "Mean Cal\n(default = ON)"() -> (w822:bool)
        n186 = local read "MFC_2 SLPM set value"() -> (w841:dbl)
        n187 = local read "MFC_3 SLPM set value"() -> (w840:dbl)
        n188 = local read "Auto Zeroing"() -> (w808:bool)
        n189 = Greater?(x=w886, y=w888) -> (0:w881:bool)
        n190 = Greater?(x=w884, y=w887) -> (0:w880:bool)
        n191 = local read "ev8 user set time"() -> (w811:i32)
        n192 = Boolean To (0,1)(Boolean=w881) -> (0, 1=w883:i16)
        n193 = Boolean To (0,1)(Boolean=w880) -> (0, 1=w882:i16)
        n194 = call "MFC_Data_Process.vi"("MFC"=w869) -> ("MFC Absolute Pressure"=w768:string, "MFC Temperature"=w767:string, "MFC Volumetric Flow"=w766:string, "MFC Mass Flow"=w765:string, "MFC Set Point"=w764:string)  [unwired: 10 in]
        n195 = call "MFC_Data_Process.vi"("MFC"=w868) -> ("MFC Absolute Pressure"=w763:string, "MFC Temperature"=w762:string, "MFC Volumetric Flow"=w761:string, "MFC Mass Flow"=w760:string, "MFC Set Point"=w759:string)  [unwired: 10 in]
        n196 = local read "ev8 zero interval"() -> (w807:i32)
        n197 = To Unsigned Long Integer(number=w883) -> (unsigned 32bit integer=w879:u32)
        n198 = To Unsigned Long Integer(number=w882) -> (unsigned 32bit integer=w878:u32)
        n199 = Number To Fractional String(number=w886, precision (6)=i16 5) -> (F-format string=w773:string)  [unwired: 2 in]
        n200 = Number To Fractional String(number=w884, precision (6)=i16 5) -> (F-format string=w772:string)  [unwired: 2 in]
        n201 = Array To Spreadsheet String(delimiter (Tab)=",", array=w800, 3:"%s" ("format string")) -> (spreadsheet string=w799:string)
        n202 = Replace Array Subset(array=w877, new element=w929, index=w876) -> (w872:string[])
        "Data Array TCP" <- w872
        n203 = Boolean To (0,1)(Boolean=w808) -> (0, 1=w810:i16)
        n204 = Boolean To (0,1)(Boolean=w779) -> (0, 1=w806:i16)
        n205 = case shown="False" w822 {
          tunnel: [w1015 w1016] -> w819
          frame False {
            n206 = local read "Zero"() -> (w1015:dbl)
          }
          frame True {
            n207 = local read "Mean Cal Offset"() -> (w1016:dbl)
          }
        }
        n208 = call <vilib>:"Trim Whitespace.vi"("string"=w799) -> ("trimmed string"=w748:string)  [unwired: 1 in]
        n209 = To Unsigned Long Integer(number=w810) -> (unsigned 32bit integer=w809:u32)
        n210 = To Unsigned Long Integer(number=w806) -> (unsigned 32bit integer=w805:u32)
        n211 = Index Array(array=w872, index=0) -> (element=w825:string)
        n212 = Concatenate Strings(w909, w915, "\r") -> ()  [unwired: 1 out]
        n213 = Number To Fractional String(number=w840, precision (6)=i16 2) -> (F-format string=w756:string)  [unwired: 2 in]
        n214 = Number To Decimal String(number=w879) -> (decimal integer string=w771:string)  [unwired: 1 in]
        n215 = Number To Decimal String(number=w878) -> (decimal integer string=w770:string)  [unwired: 1 in]
        n216 = Number To Fractional String(number=w841, precision (6)=i16 2) -> (F-format string=w757:string)  [unwired: 2 in]
        n217 = Number To Decimal String(number=w811) -> (decimal integer string=w752:string)  [unwired: 1 in]
        n218 = Number To Decimal String(number=w809, width (-)=i16 1) -> (decimal integer string=w751:string)
        n219 = Number To Decimal String(number=w807) -> (decimal integer string=w750:string)  [unwired: 1 in]
        n220 = Number To Decimal String(number=w805, width (-)=i16 1) -> (decimal integer string=w749:string)
        n221 = Boolean To (0,1)(Boolean=w789) -> (0, 1=w791:i16)
        n222 = local read "Slope"() -> (w818:dbl)
        n223 = Boolean To (0,1)(Boolean=w822) -> (0, 1=w824:i16)
        n224 = local read "Flight Number"() -> (w775:string)
        n225 = To Unsigned Long Integer(number=w791) -> (unsigned 32bit integer=w790:u32)
        n226 = Number To Fractional String(number=w818, precision (6)=i16 2) -> (F-format string=w753:string)  [unwired: 2 in]
        n227 = Number To Decimal String(number=w824, width (-)=i16 1) -> (decimal integer string=w755:string)
        n228 = Number To Fractional String(number=w819, precision (6)=i16 2) -> (F-format string=w754:string)  [unwired: 2 in]
        n229 = Scan From String(format string="%f", input string=w825) -> (output 1=w829:dbl)  [unwired: 3 in, 3 out]
        n230 = Number To Decimal String(number=w790) -> (decimal integer string=w746:string)  [unwired: 1 in]
        n231 = Number To Fractional String(number=w787, precision (6)=i16 2) -> (F-format string=w745:string)  [unwired: 2 in]
        n232 = call "SO2 Calibration Equation.vi"("Input"=w829, "Offset"=w819, "Slope"=w818) -> ("Output"=w815:dbl)  [unwired: 12 in]
        n233 = case shown="True" w779 {
          tunnel: w817 -> [_ w988]
          tunnel: [0 w986] -> w816
          tunnel: w789 -> [_ w991]
          tunnel: w787 -> [_ w990]
          tunnel: w815 -> [_ w989]
          tunnel: [FALSE w987] -> w812
          tunnel: w778 -> [_ w985]
          frame False {
          }
          frame True {
            # "MOCCA SO2 alarm"
            n234 = case shown="True" w985 {
              tunnel: w991 -> [_ w1001]
              tunnel: w990 -> [_ w1000]
              tunnel: w989 -> [_ w999]
              tunnel: w988 -> [w993 w998]
              tunnel: [w992 w996] -> w987
              tunnel: [w993 w995] -> w986
              frame False {
                n235 = local read "local\ndummy"() -> (w992:bool)
              }
              frame True {
                # "check every 1 second"
                n236 = local read "MOCCA window delay time (sec)"() -> (w997:i32)
                n237 = Select(t=w1000, s=w1001, f=w999) -> (s? t:f=w1002:dbl)
                n238 = local read "MOCCA SO2 Limit"() -> (w1003:i32)
                n239 = To Long Integer(number=w1002) -> (32bit integer=w1004:i32)
                n240 = Greater Or Equal?(x=w1004, y=w1003) -> (x >= y?=w994:bool)
                n241 = case shown="True" w994 {
                  tunnel: w998 -> [_ w1010]
                  tunnel: w997 -> [_ w1009]
                  tunnel: [FALSE w1008] -> w996
                  tunnel: [0 w1007] -> w995
                  frame False {
                  }
                  frame True {
                    n242 = Increment(x=w1010) -> (x+1=w1007:i32)
                    n243 = Greater?(x=w1007, y=w1009) -> (0:w1008:bool)
                  }
                }
                "local\ndummy" <- w996
              }
            }
          }
        }
        n244 = case shown="True" w778 {
          tunnel: w891 -> [_ w1064]
          tunnel: w815 -> [_ w1061]
          tunnel: w815 -> [_ w1063]
          tunnel: w890 -> [_ w1062]
          tunnel: w831 -> [_ w1057]
          tunnel: w830 -> [w1048 w1056]
          tunnel: w829 -> [_ w1054]
          tunnel: [w1048 w1052] -> w828
          tunnel: w827 -> [w1047 w1051]
          tunnel: [w1047 w1050] -> w826
          frame False {
          }
          frame True {
            w1049 = 5 ("y")
            # "Mean offset calculation - 5 secs after ev8 is turned ON"
            # "SO2 monitor every second"
            n245 = Equal?(x=w1057, y=TRUE) -> (x = y?=w1059:bool)
            n246 = Increment(x=w1056) -> (x+1=w1058:i32)
            n247 = Select(t=w1058, s=w1059, f=0) -> (s? t:f=w1052:i32)
            n248 = Greater?(x=w1052, y=w1049) -> (0:w1055:bool)
            n249 = case shown="True" w1055 {
              tunnel: w1054 -> [_ w1070]
              tunnel: [w1065 w1069] -> w1050
              tunnel: w1051 -> [w1065 _]
              tunnel: w1049 -> [_ w1068]
              frame False {
              }
              frame True {
                n250 = local read "ev8 user set time"() -> (w1066:i32)
                n251 = Subtract(x=w1066, y=w1068) -> (x-y=w1067:i32)
                n252 = call <vilib>:"Mean PtByPt.vi"("x"=w1070, "sample length"=w1067) -> ("mean"=w1069:dbl)  [unwired: 2 in, 1 out]
              }
            }
            "Mean Cal Offset" <- w1050
            n253 = Lossy Enqueue Element(queue=w1064, element=w1061) -> ()  [unwired: 1 in, 4 out]
            n254 = Lossy Enqueue Element(queue=w1062, element=w1063) -> ()  [unwired: 1 in, 4 out]
          }
        }
        n255 = Boolean To (0,1)(Boolean=w812) -> (0, 1=w814:i16)
        n256 = To Unsigned Long Integer(number=w814) -> (unsigned 32bit integer=w813:u32)
        n257 = Number To Decimal String(number=w813, width (-)=i16 1) -> (decimal integer string=w743:string)
        n258 = case shown="True" "Clear Display\nErrors" {
          frame False {
          }
          frame True {
            w1071 = errorcluster {"status"=FALSE, "code"=0, "source"=""} ("UDP Error Out")
            n259 = local write "SEPTIC TCP Error Out"(w1071) -> ()
            n260 = local write "Serial Visa Error"(w1071) -> ()
            n261 = local write "FISH TCP Error Out"(w1071) -> ()
            n262 = local write "UDP_Out_Error"(w1071) -> ()
          }
        }
        n263 = Number To Fractional String(number=w815, precision (6)=i16 5) -> (F-format string=w873:string)  [unwired: 2 in]
        n264 = Replace Array Subset(array=w872, new element=w873, index=0) -> (w871:string[])
        "Data Array UDP" <- w871
        n265 = Array To Spreadsheet String(delimiter (Tab)=",", array=w871, 3:"%s" ("format string")) -> (spreadsheet string=w925:string)
        n266 = call <vilib>:"Trim Whitespace.vi"("string"=w925, "location (both)"=w926) -> ("trimmed string"=w774:string)
        "Data String" <- w774
        n267 = Concatenate Strings(w898, w786, w777, w786, w769, w786, w775, w786, w834, w786, w833, w786, w774, w786, w773, w786, w772, w786, w771, w786, w770, w786, w768, w786, w767, w786, w766, w786, w765, w786, w764, w786, w763, w786, w762, w786, w761, w786, w760, w786, w759, w786, w758, w786, w757, w786, w756, w786, w825, w786, w755, w786, w754, w786, w753, w786, w752, w786, w751, w786, w750, w786, w749, w786, w748, w786, w747, w786, w746, w786, w745, w786, w743) -> (w931:string)
        n268 = Concatenate Strings(w777, w744, "dummy", w744, w775, w744, w769, w744, w773, w744, w772, w744, w771, w744, w770, w744, w768, w744, w767, w744, w766, w744, w765, w744, w764, w744, w763, w744, w762, w744, w761, w744, w760, w744, w759, w744, w758, w744, w757, w744, w756, w744, w755, w744, w754, w744, w753, w744, w752, w744, w751, w744, w750, w744, w749, w744, w748, w744, w747, w744, w746, w744, w745, w744, w743) -> (w742:string)
        n269 = local read "Stop File Write"() -> (w856:bool)
        n270 = call "SO2 TCP Packet_v3.1.vi"("ID"=w741, "Version"=w740, "TCP Packet In"=w742, "utc_time"=w739, "Data Array"=w872) -> ("TCP Binary Packet"=w900:string)  [unwired: 10 in]
        "TCP Binary Packet" <- w900
        n271 = String Length(string=w931) -> (length=w935:i32)
        n272 = Enqueue Element(queue=w902, element=w900, error in (no error)=w901) -> ()  [unwired: 1 in, 3 out]
        n273 = Enqueue Element(queue=w914, element=w900, error in (no error)=w913) -> ()  [unwired: 1 in, 3 out]
        n274 = Number To Decimal String(number=w935, width (-)=i16 3) -> (decimal integer string=w933:string)
        n275 = Concatenate Strings(w741, w740, w932, w933, w932, w931) -> (w857:string)
        "UDP_ASCII_Out" <- w857
        n276 = case shown="False" w856 {
          tunnel: w857 -> [w1042 _]
          tunnel: w864 -> [w1044 w1046]
          tunnel: w863 -> [w1043 w1045]
          tunnel: [w1039 _] -> w859
          tunnel: [w1038 _] -> w858
          frame False {
            n277 = Concatenate Strings(w1042, "\r") -> (w1040:string)
            n278 = Write to Text File(file (use dialog)=w1044, text=w1040, error in=w1043) -> (refnum out=w1039:refnum<file>, error out=w1038:errorcluster)  [unwired: 2 out]
          }
          frame True {
            n279 = Close File(refnum=w1046, error in=w1045) -> ()  [unwired: 2 out]
          }
        }
        n280 = case shown="True" w778 {
          tunnel: w912 -> [_ w1074]
          tunnel: w911 -> [_ w1073]
          tunnel: w857 -> [_ w1072]
          frame False {
          }
          frame True {
            # "Send UDP data once\na second"
            n281 = Enqueue Element(queue=w1074, element=w1072, error in (no error)=w1073) -> ()  [unwired: 1 in, 3 out]
          }
        }
        n282 = local read "stop"() -> (w938:bool)
        n283 = node-c288() -> ()  [unwired: 1 in, 1 out]
      }
      n284 = node-c288() -> (w84:T4)  [unwired: 4 in]
      n285 = node-c288() -> (w86:T4)  [unwired: 4 in]
      n286 = timed-loop {
        tunnel: w90 -> [w423]
        timing: w84 -> [_]
        timing-out: [_] -> w83
        stop <- w424 stop-if-true
        # "10 minutes SO2 Average calculated every second"
        n287 = node-c288() -> ()  [unwired: 1 in, 1 out]
        n288 = Get Queue Status(queue=w423, return elements? (F)=TRUE) -> (elements=w414:dbl[])  [unwired: 1 in, 7 out]
        n289 = for {
          tunnel: w414 -> [w427] mode=indexing
          tunnel: [w431] -> w420
          shift-right: [w430] -> w418
          shift-left: i64 0 -> [w429]
          i -> [w431]
          n290 = To Quad Integer(1:w427) -> (0:w428:i64)
          n291 = Add(x=w429, y=w428) -> (x+y=w430:i64)
        }
        n292 = Increment(x=w420) -> (x+1=w415:i32)
        "q_size" <- w415
        n293 = To Double Precision Float(number=w418) -> (double precision float=w416:dbl)
        n294 = To Double Precision Float(number=w415) -> (double precision float=w417:dbl)
        n295 = Divide(x=w416, y=w417) -> (x/y=→"10min_so2_avg":dbl)
        n296 = local read "stop"() -> (w424:bool)
        n297 = node-c288() -> ()  [unwired: 1 in, 1 out]
      }
      n298 = timed-loop {
        tunnel: w89 -> [w443]
        timing: w86 -> [_]
        timing-out: [_] -> w85
        stop <- w444 stop-if-true
        # "8 hours SO2 Average calculated every second"
        n299 = node-c288() -> ()  [unwired: 1 in, 1 out]
        n300 = Get Queue Status(queue=w443, return elements? (F)=TRUE) -> (elements=w440:dbl[])  [unwired: 1 in, 7 out]
        n301 = for {
          tunnel: w440 -> [w447] mode=indexing
          tunnel: [w451] -> w439
          shift-right: [w450] -> w437
          shift-left: i64 0 -> [w449]
          i -> [w451]
          n302 = To Quad Integer(1:w447) -> (0:w448:i64)
          n303 = Add(x=w449, y=w448) -> (x+y=w450:i64)
        }
        n304 = Increment(x=w439) -> (x+1=w434:i32)
        "q_size 2" <- w434
        n305 = To Double Precision Float(number=w437) -> (double precision float=w435:dbl)
        n306 = To Double Precision Float(number=w434) -> (double precision float=w436:dbl)
        n307 = Divide(x=w435, y=w436) -> (x/y=→"8hr_so2_avg 2":dbl)
        n308 = local read "stop"() -> (w444:bool)
        n309 = node-c288() -> ()  [unwired: 1 in, 1 out]
      }
      n310 = while {
        tunnel: [w598] -> w112
        tunnel: w82 -> [w611]
        tunnel: w81 -> [w610]
        tunnel: [w609] -> w111
        tunnel: w108 -> [w608]
        shift-right: [w606] -> _
        shift-left: 0 -> [w607]
        shift-right: [w604] -> _
        shift-left: u32 0 -> [w605]
        tunnel: w93 -> [w596]
        stop <- "stop" stop-if-true
        w599 = 2
        w601 = string[] ["pmt voltage", "lamp voltage", "lamp int", "internal temp", "react temp", "pres", "flow", "flags"]
        # ">>Monitor command enter as a pair>>"
        # ">>Main commands>>"
        # ">>Monitor Command>>"
        n311 = Array Size(array=w601) -> (size(s)=w602:i32)
        n312 = Divide(x=w602, y=w599) -> (x/y=w600:dbl)
        n313 = for {
          N: w600 -> [_]
          tunnel: w611 -> [w621]
          tunnel: w610 -> [w620]
          tunnel: [w630] -> w598
          shift-right: [w628] -> w606
          shift-left: w607 -> [w629]
          shift-right: [w626] -> w604
          shift-left: w605 -> [w627]
          tunnel: [w625] -> w609
          tunnel: w608 -> [w624]
          tunnel: w601 -> [w617]
          tunnel: "so2" -> [w622]
          tunnel: w599 -> [w618]
          tunnel: w596 -> [w612]
          i -> [w619]
          # "FOR Loop runs according\nto the number of monitor commands"
          # "Assemble command:\nso2\npmt voltage\nlamp voltage\n\netc\netc\n\nso2\nflow\nflags"
          n314 = Multiply(x=w618, y=w619) -> (x*y=w615:i32)
          n315 = Array Subset(array=w617, index=w615, length=w618) -> (w616:string[])
          n316 = Build Array (concatenate)(w622, w616) -> (w623:string[])
          "Data In Array" <- w623
          n317 = node-c288() -> (w614:T4)  [unwired: 4 in]
          n318 = timed-sequence {
            timing: w614 -> [_]
            timing-out: [_] -> w613
            tunnel: w629 -> [w652]
            tunnel: w623 -> [w651]
            tunnel: w621 -> [w650]
            tunnel: w620 -> [w649]
            tunnel: w615 -> [w648]
            tunnel: w624 -> [w643]
            tunnel: [w639] -> w630
            tunnel: [w637] -> w628
            tunnel: w627 -> [w635]
            tunnel: [w634] -> w626
            tunnel: [w633] -> w625
            tunnel: w612 -> [w631]
            n319 = timed-flat-sequence {
              tunnel: w651 -> [w657]
              tunnel: w652 -> [w658]
              tunnel: [w655] -> w647
              tunnel: [w658] -> w646
              tunnel: [w657] -> w645
              tunnel: [w656] -> w644
              tunnel: w650 -> [w655]
              tunnel: [w654] -> w642
              tunnel: w649 -> [w654]
              tunnel: [w653] -> w641
              tunnel: w648 -> [w653]
              tunnel: [w671] -> w640
              tunnel: [w668] -> w638
              tunnel: w647 -> [w663]
              tunnel: w646 -> [w670]
              tunnel: w645 -> [w669]
              tunnel: [w667] -> w636
              tunnel: w644 -> [w667]
              tunnel: [w666] -> w632
              tunnel: w643 -> [w665]
              tunnel: w642 -> [w664]
              tunnel: w641 -> [w662]
              tunnel: w631 -> [w661]
              tunnel: [w733] -> w637
              tunnel: [w734] -> w639
              tunnel: w640 -> [w734]
              tunnel: w638 -> [w733]
              tunnel: w636 -> [w729]
              tunnel: w635 -> [w728]
              tunnel: [w727] -> w634
              tunnel: [w726] -> w633
              tunnel: w632 -> [w726]
              frame #0 {
                n320 = node-c288() -> ()  [unwired: 1 in, 1 out]
                n321 = node-c288() -> ()  [unwired: 1 in, 1 out]
                n322 = Tick Count (ms)() -> (millisecond timer value=w656:u32)
              }
              frame #1 {
                n323 = node-c288() -> ()  [unwired: 1 in, 1 out]
                n324 = while {
                  tunnel: [w685] -> w671
                  tunnel: w669 -> [w683]
                  tunnel: [w681] -> w666
                  tunnel: w665 -> [w680]
                  tunnel: w664 -> [w679]
                  tunnel: w663 -> [w678]
                  tunnel: w662 -> [w677]
                  shift-right: [w682] -> w668
                  shift-left: w670 -> [w684]
                  tunnel: w661 -> [w674]
                  stop <- TRUE stop-if-true
                  # "Receive data is organised as:\nDate Time so2 DATA -1\nDate Time pmt voltage DATA 0\nDate Time lamp voltage DATA 1\nDate Time so2 DATA -1\nDate Time lamp int DATA 2\nDate Time internal temp DATA 3\nDate Time so2 DATA -1\nDate Time react temp DATA 4\nDate Time pres DATA 5\nDate Time so2 DATA -1\nDate Time flow DATA 6\nDate Time flags DATA 7\n\nDate Time Read Error -2"
                  n325 = for {
                    tunnel: w679 -> [w702]
                    tunnel: [w703] -> w685
                    tunnel: w683 -> [w700] mode=indexing
                    tunnel: [w704] -> w681
                    tunnel: w680 -> [w710]
                    tunnel: w678 -> [w705]
                    tunnel: w677 -> [w699]
                    shift-right: [w714] -> w682
                    shift-left: w684 -> [w715]
                    tunnel: w674 -> [w688]
                    i -> [w692]
                    # "Acquire every 330msec for 3 times\nto make 1 second"
                    # "SO2 Acquisition Loop"
                    n326 = call "Wait"("Count(mSec)"=w688) -> ()  [unwired: 1 out]
                    n327 = Concatenate Strings("ID", w700, "\r") -> (w698:string)
                    "Command In" <- w698
                    n328 = call "SO2 Serial Packet Write.vi"("VISA resource name In"=w705, "Data in"=w698, "error in (no error)"=w702) -> ("VISA resource name Out"=w707:refnum<visa-resource-name>, "error out"=w706:errorcluster)  [unwired: 11 in]
                    n329 = call "SO2 Serial Packet Read.vi"("VISA resource In"=w707, "error in"=w706) -> ("VISA resource Out"=w704:refnum<visa-resource-name>, "Data Out"=w695:string, "error out"=w703:errorcluster)  [unwired: 11 in]
                    "RAW DATA" <- w695
                    n330 = Equal?(x=w695, y="Read Error") -> (x = y?=w693:bool)
                    n331 = Get Date/Time In Seconds() -> (seconds since 1Jan1904=w687:timestamp)
                    n332 = case shown="False" w693 {
                      tunnel: [w718 "-2"] -> w708
                      tunnel: w692 -> [w717 _]
                      tunnel: w699 -> [w716 _]
                      frame False {
                        n333 = case shown="0" w717 {
                          tunnel: ["-1" w722 w724] -> w718
                          tunnel: w716 -> [_ w720 w723]
                          frame 0 {
                            # "Make internal flag\n-1 represent so2 data"
                          }
                          frame 2 {
                            # "Make internal flag"
                            n334 = Increment(x=w720) -> (x+1=w721:i32)
                            n335 = Number To Decimal String(number=w721) -> (decimal integer string=w722:string)  [unwired: 1 in]
                          }
                          frame 1, Default {
                            # "Make internal flag"
                            n336 = Number To Decimal String(number=w723) -> (decimal integer string=w724:string)  [unwired: 1 in]
                          }
                        }
                      }
                      frame True {
                      }
                    }
                    n337 = Increment(x=w715) -> (x+1=w711:i32)
                    n338 = Unbundle(w703) -> ("status"=w712:bool)  [unwired: 2 out]
                    n339 = call <vilib>:"Trim Whitespace.vi"("string"=w695) -> ("trimmed string"=w709:string)  [unwired: 1 in]
                    n340 = To Unsigned Long Integer(number=w687) -> (unsigned 32bit integer=w691:u32)
                    n341 = Subtract(x=w691, y=u32 2082844800) -> (x-y=w686:u32)
                    n342 = Select(t=w711, s=w712, f=w715) -> (s? t:f=w714:i32)
                    n343 = call <vilib>:"Space Constant.vi"() -> ("String"=w696:string)
                    n344 = Number To Decimal String(number=w686) -> (decimal integer string=w689:string)  [unwired: 1 in]
                    n345 = Build Array(w689, w696, w709, w696, w708) -> (w697:string[])
                    n346 = Enqueue Element(queue=w710, element=w697) -> ()  [unwired: 2 in, 3 out]
                  }
                  "Number of Send & Read Error\nfrom Acquire Loop" <- w682
                  n347 = call "Wait Until Next Multiple"("Count(mSec)"=u32 1000) -> ()  [unwired: 1 out]
                }
                n348 = node-c288() -> ()  [unwired: 1 in, 1 out]
              }
              frame #2 {
                n349 = node-c288() -> ()  [unwired: 1 in, 1 out]
                n350 = Tick Count (ms)() -> (millisecond timer value=w732:u32)
                n351 = Subtract(x=w732, y=w729) -> (x-y=w731:u32)
                "Acq Time" <- w731
                "Time taken history" <- w731
                n352 = Greater?(x=w731, y=w728) -> (0:w730:bool)
                n353 = Select(t=w731, s=w730, f=w728) -> (s? t:f=w727:u32)
                "Max Acq Time diff" <- w727
                n354 = node-c288() -> ()  [unwired: 1 in, 1 out]
              }
            }
          }
          n355 = node-c288(w613) -> ()  [unwired: 1 out]
        }
      }
      n356 = node-c288(w85) -> ()  [unwired: 1 out]
      n357 = node-c288(w83) -> ()  [unwired: 1 out]
      n358 = while {
        stop <- FALSE stop-if-true
        # "CAL MFC 3 status & control"
        n359 = Wait (ms)(milliseconds to wait=u32 1000) -> ()  [unwired: 1 out]
        n360 = call-poly "VISA Configure Serial Port"("VISA resource name"="VISA resource name 2", "timeout (10sec)"="timeout (10sec) 2", "termination char\n(0xA = '\\n' = LF)"=u8 13 ("termination char\n(0xA = '\\n' = LF)"), "Enable Termination\nChar (T)"=TRUE ("Enable Termination\nChar (T)"), "baud rate (9600)"=u32 19200) -> ("VISA resource name out"=w355:refnum<visa-resource-name>, "error out"=w351:errorcluster)  [unwired: 9 in]
        n361 = case shown="No Error" w351 {
          selector: w351 -> [w362 w412]
          tunnel: w355 -> [w363 w413]
          tunnel: [w361 w413] -> w354
          tunnel: [w360 w412] -> w353
          frame No Error {
            n362 = node-c288() -> (w358:T4)  [unwired: 4 in]
            n363 = timed-loop {
              tunnel: w363 -> [w386]
              tunnel: w362 -> [w384]
              tunnel: [w377] -> w361
              tunnel: [w372] -> w360
              shift-right: [w373] -> _
              shift-left: FALSE -> [w376]
              timing: w358 -> [_]
              timing-out: [_] -> w357
              shift-right: [w364] -> _
              shift-left: 0.0 -> [w366]
              stop <- w372 stop-if-true
              n364 = node-c288() -> ()  [unwired: 1 in, 1 out]
              n365 = local read "MFC_3 SLPM set value"() -> (w364:dbl)
              n366 = Not Equal?(x=w364, y=w366) -> (x != y?=w365:bool)
              n367 = case shown="True" w365 {
                tunnel: w386 -> [w394 w409]
                tunnel: [w394 w409] -> w385
                tunnel: w384 -> [w393 w408]
                tunnel: [w393 w408] -> w383
                tunnel: "A" -> [w397 w401]
                tunnel: [w395 w398] -> w381
                frame False {
                  n368 = Concatenate Strings(w397, "\r") -> (w395:string)
                }
                frame True {
                  n369 = Multiply(x="MFC_3 SLPM set value", y=u32 64000) -> (x*y=w405:dbl)
                  n370 = Divide(x=w405, y=u32 5) -> (x/y=w403:dbl)
                  n371 = To Unsigned Long Integer(number=w403) -> (unsigned 32bit integer=w402:u32)
                  n372 = Number To Decimal String(number=w402) -> (decimal integer string=w400:string)  [unwired: 1 in]
                  n373 = Concatenate Strings(w401, w400, "\r") -> (w398:string)
                }
              }
              n374 = VISA Flush I/O Buffer(VISA resource name=w385, error in (no error)=w383) -> (VISA resource name out=w388:refnum<visa-resource-name>, error out=w387:errorcluster)  [unwired: 1 in]
              n375 = Select(t=FALSE, s=w376, f=TRUE) -> (s? t:f=w373:bool)
              "status" <- w373
              n376 = VISA Write(VISA resource name=w388, write buffer=w381, error in (no error)=w387) -> (VISA resource name out=w380:refnum<visa-resource-name>, error out=w379:errorcluster)  [unwired: 1 out]
              n377 = VISA Flush I/O Buffer(VISA resource name=w380, error in (no error)=w379) -> (VISA resource name out=w390:refnum<visa-resource-name>, error out=w389:errorcluster)  [unwired: 1 in]
              n378 = VISA Read(VISA resource name=w390, byte count=u32 50, error in (no error)=w389) -> (VISA resource name out=w377:refnum<visa-resource-name>, read buffer=w371:string, error out=w372:errorcluster)  [unwired: 1 out]
              "Value Read 3" <- w371
              n379 = call <vilib>:"Space Constant.vi"() -> ("String"=w370:string)
              n380 = Spreadsheet String To Array(delimiter (Tab)=w370, format string="%f", spreadsheet string=w371, array type (2D Dbl)=dbl[] []) -> (array=→"MFC 3":dbl[])
              n381 = node-c288() -> ()  [unwired: 1 in, 1 out]
            }
            n382 = node-c288(w357) -> ()  [unwired: 1 out]
          }
          frame Error {
          }
        }
        n383 = VISA Close(VISA resource name=w354, error in (no error)=w353) -> (error out=→"error out 3":errorcluster)
      }
      n384 = while {
        stop <- FALSE stop-if-true
        # "CAL MFC 2 status & control"
        n385 = Wait (ms)(milliseconds to wait=u32 1000) -> ()  [unwired: 1 out]
        n386 = call-poly "VISA Configure Serial Port"("VISA resource name"="VISA resource name 3", "timeout (10sec)"="timeout (10sec) 3", "termination char\n(0xA = '\\n' = LF)"=u8 13 ("termination char\n(0xA = '\\n' = LF)"), "Enable Termination\nChar (T)"=TRUE ("Enable Termination\nChar (T)"), "baud rate (9600)"=u32 19200) -> ("VISA resource name out"=w285:refnum<visa-resource-name>, "error out"=w281:errorcluster)  [unwired: 9 in]
        n387 = case shown="No Error" w281 {
          selector: w281 -> [w292 w342]
          tunnel: w285 -> [w293 w343]
          tunnel: [w291 w343] -> w284
          tunnel: [w290 w342] -> w283
          frame No Error {
            n388 = node-c288() -> (w288:T4)  [unwired: 4 in]
            n389 = timed-loop {
              tunnel: w293 -> [w316]
              tunnel: w292 -> [w314]
              tunnel: [w307] -> w291
              tunnel: [w302] -> w290
              shift-right: [w303] -> _
              shift-left: FALSE -> [w306]
              timing: w288 -> [_]
              timing-out: [_] -> w287
              shift-right: [w294] -> _
              shift-left: 0.0 -> [w296]
              stop <- w302 stop-if-true
              n390 = node-c288() -> ()  [unwired: 1 in, 1 out]
              n391 = local read "MFC_2 SLPM set value"() -> (w294:dbl)
              n392 = Not Equal?(x=w294, y=w296) -> (x != y?=w295:bool)
              n393 = case shown="True" w295 {
                tunnel: w316 -> [w324 w339]
                tunnel: [w324 w339] -> w315
                tunnel: w314 -> [w323 w338]
                tunnel: [w323 w338] -> w313
                tunnel: "A" -> [w327 w331]
                tunnel: [w325 w328] -> w311
                frame False {
                  n394 = Concatenate Strings(w327, "\r") -> (w325:string)
                }
                frame True {
                  n395 = Multiply(x="MFC_2 SLPM set value", y=u32 64000) -> (x*y=w335:dbl)
                  n396 = Divide(x=w335, y=u32 5) -> (x/y=w333:dbl)
                  n397 = To Unsigned Long Integer(number=w333) -> (unsigned 32bit integer=w332:u32)
                  n398 = Number To Decimal String(number=w332) -> (decimal integer string=w330:string)  [unwired: 1 in]
                  n399 = Concatenate Strings(w331, w330, "\r") -> (w328:string)
                }
              }
              n400 = Select(t=FALSE, s=w306, f=TRUE) -> (s? t:f=w303:bool)
              "status 2" <- w303
              n401 = VISA Flush I/O Buffer(VISA resource name=w315, error in (no error)=w313) -> (VISA resource name out=w318:refnum<visa-resource-name>, error out=w317:errorcluster)  [unwired: 1 in]
              n402 = VISA Write(VISA resource name=w318, write buffer=w311, error in (no error)=w317) -> (VISA resource name out=w310:refnum<visa-resource-name>, error out=w309:errorcluster)  [unwired: 1 out]
              n403 = VISA Flush I/O Buffer(VISA resource name=w310, error in (no error)=w309) -> (VISA resource name out=w320:refnum<visa-resource-name>, error out=w319:errorcluster)  [unwired: 1 in]
              n404 = VISA Read(VISA resource name=w320, byte count=u32 50, error in (no error)=w319) -> (VISA resource name out=w307:refnum<visa-resource-name>, read buffer=w301:string, error out=w302:errorcluster)  [unwired: 1 out]
              "Value Read 2" <- w301
              n405 = call <vilib>:"Space Constant.vi"() -> ("String"=w300:string)
              n406 = Spreadsheet String To Array(delimiter (Tab)=w300, format string="%f", spreadsheet string=w301, array type (2D Dbl)=dbl[] []) -> (array=→"MFC 2":dbl[])
              n407 = node-c288() -> ()  [unwired: 1 in, 1 out]
            }
            n408 = node-c288(w287) -> ()  [unwired: 1 out]
          }
          frame Error {
          }
        }
        n409 = VISA Close(VISA resource name=w284, error in (no error)=w283) -> (error out=→"error out 2":errorcluster)
      }
      n410 = node-c288(w109) -> ()  [unwired: 1 out]
      n411 = while {
        stop <- FALSE stop-if-true
        n412 = node-c288() -> (w114:T4)  [unwired: 4 in]
        n413 = Create Network Stream Reader Endpoint(7:10 ("reader buffer size"), 9:T3 {"Message"="", "Message Data"=variant} ("Message Cluster"), 11:"/command/reader/SO2" ("reader url")) -> (0:w120:errorcluster, 3:w121:refnum<k21>)  [unwired: 4 in]
        n414 = timed-loop "Host->Target Command Reader" {
          shift-right: [w131] -> w118
          shift-left: w120 -> [w134]
          shift-right: [w132] -> w117
          shift-left: w121 -> [w133]
          tunnel: [TRUE] -> _
          timing: w114 -> [_]
          timing-out: [_] -> w113
          stop <- w125 stop-if-true
          # "Receive Commands from Host VI"
          n415 = node-c288() -> ()  [unwired: 1 in, 1 out]
          n416 = shared-variable-read(w133, w134) -> (w132:refnum<k21>, w127:errorcluster, w129:bool, w130:T3)  [unwired: 1 in]
          n417 = Or(x=w129, y=w127) -> (x .or. y?=w128:bool)
          n418 = case shown="False" w128 {
            selector: w128 -> [_ w270]
            tunnel: w127 -> [w142 w271]
            tunnel: [w141 w271] -> w131
            tunnel: w130 -> [w139 _]
            tunnel: [w140 w270] -> w125
            frame False {
              n419 = Unbundle By Name(w139) -> ("Message"=w138:string, "Message Data"=w137:variant)
              n420 = case shown="\"zeroing_interval\"" w138 {
                tunnel: w142 -> [w144 w149 w154 w159 w164 w169 w174 w179 w184 w189 w194 w199 w204 w209 w214 w219 w224 w229 w234 w239 w244 w249 w254 w258 w263 w268]
                tunnel: [w144 w148 w153 w158 w163 w168 w173 w178 w183 w188 w193 w198 w203 w208 w213 w218 w223 w228 w233 w238 w243 w248 w253 w256 w261 w266] -> w141
                tunnel: w137 -> [_ w147 w152 w157 w162 w167 w172 w177 w182 w187 w192 w197 w202 w207 w212 w217 w222 w227 w232 w237 w242 w247 w252 w259 w264 w269]
                tunnel: [TRUE _ _ _ _ _ _ _ _ _ _ _ _ _ _ _ _ _ _ _ _ _ _ _ _ _] -> w140
                frame "Stop", Default {
                }
                frame "V9" {
                  n421 = Variant To Data(error in=w149, type=FALSE, Variant=w147) -> (data=w145:bool, error out=w148:errorcluster)
                  "V9" <- w145
                  n422 = shared-variable "NI-cRIO9022-019C2C95\\Mod6\\DO7"(w145) -> ()  [unwired: 1 in, 1 out]
                }
                frame "MFC_2" {
                  n423 = Variant To Data(error in=w154, type=0.0, Variant=w152) -> (data=w150:dbl, error out=w153:errorcluster)
                  n424 = local write "MFC_2 SLPM set value"(w150) -> ()
                }
                frame "cal_gas_cylin_conc" {
                  n425 = Variant To Data(error in=w159, type=0.0, Variant=w157) -> (data=→"cal gas cylinder conc":dbl, error out=w158:errorcluster)
                }
                frame "sim_MOCCA_conc" {
                  n426 = Variant To Data(error in=w164, type=0.0, Variant=w162) -> (data=→"Simulate MOCCA Conc":dbl, error out=w163:errorcluster)
                }
                frame "Auto_zero" {
                  n427 = Variant To Data(error in=w169, type=FALSE, Variant=w167) -> (data=→"Auto Zeroing":bool, error out=w168:errorcluster)
                }
                frame "zeroing_interval" {
                  n428 = Variant To Data(error in=w174, type=0, Variant=w172) -> (data=→"ev8 zero interval":i32, error out=w173:errorcluster)
                }
                frame "MOCCA_window_delay_time" {
                  n429 = Variant To Data(error in=w179, type=0, Variant=w177) -> (data=→"MOCCA window delay time (sec)":i32, error out=w178:errorcluster)
                }
                frame "MOCCA_limit" {
                  n430 = Variant To Data(error in=w184, type=0, Variant=w182) -> (data=→"MOCCA SO2 Limit":i32, error out=w183:errorcluster)
                }
                frame "eV8_user_set_time" {
                  n431 = Variant To Data(error in=w189, type=0, Variant=w187) -> (data=→"ev8 user set time":i32, error out=w188:errorcluster)
                }
                frame "MFC_3" {
                  n432 = Variant To Data(error in=w194, type=0.0, Variant=w192) -> (data=w190:dbl, error out=w193:errorcluster)
                  n433 = local write "MFC_3 SLPM set value"(w190) -> ()
                }
                frame "Simulate STEL Conc" {
                  n434 = Variant To Data(error in=w199, type=0.0, Variant=w197) -> (data=→"Simulate STEL Conc":dbl, error out=w198:errorcluster)
                }
                frame "Simulate TWA Conc" {
                  n435 = Variant To Data(error in=w204, type=0.0, Variant=w202) -> (data=→"Simulate TWA Conc":dbl, error out=w203:errorcluster)
                }
                frame "Offset" {
                  n436 = Variant To Data(error in=w209, type=0.0, Variant=w207) -> (data=→"Zero":dbl, error out=w208:errorcluster)
                }
                frame "10mins STEL Limit" {
                  n437 = Variant To Data(error in=w214, type=0, Variant=w212) -> (data=→"10mins_STEL_limit":i32, error out=w213:errorcluster)
                }
                frame "UDP Time Offset" {
                  n438 = Variant To Data(error in=w219, type=0, Variant=w217) -> (data=→"UDP Time Stamp Offset":i32, error out=w218:errorcluster)
                }
                frame "8hr TWA Limit" {
                  n439 = Variant To Data(error in=w224, type=0, Variant=w222) -> (data=→"8hr_TWA_limit":i32, error out=w223:errorcluster)
                }
                frame "Slope" {
                  n440 = Variant To Data(error in=w229, type=0.0, Variant=w227) -> (data=→"Slope":dbl, error out=w228:errorcluster)
                }
                frame "V8" {
                  n441 = Variant To Data(error in=w234, type=FALSE, Variant=w232) -> (data=w230:bool, error out=w233:errorcluster)
                  "V8" <- w230
                  n442 = shared-variable "NI-cRIO9022-019C2C95\\Mod6\\DO6"(w230) -> ()  [unwired: 1 in, 1 out]
                }
                frame "Stop File Write" {
                  n443 = Variant To Data(error in=w239, type=FALSE, Variant=w237) -> (data=→"Stop File Write":bool, error out=w238:errorcluster)
                }
                frame "SO2_MOCCA_Alarm" {
                  n444 = Variant To Data(error in=w244, type=FALSE, Variant=w242) -> (data=→"SO2 Inflight MOCCA Alarm\n(default = OFF)":bool, error out=w243:errorcluster)
                }
                frame "Flight Number" {
                  n445 = Variant To Data(error in=w249, type="", Variant=w247) -> (data=→"Flight Number":string, error out=w248:errorcluster)
                }
                frame "V6" {
                  n446 = Variant To Data(error in=w254, type=FALSE, Variant=w252) -> (data=w250:bool, error out=w253:errorcluster)
                  "V6" <- w250
                  n447 = shared-variable "NI-cRIO9022-019C2C95\\Mod6\\DO4"(w250) -> ()  [unwired: 1 in, 1 out]
                }
                frame "Simulate Conc" {
                  n448 = Variant To Data(error in=w258, type=FALSE, Variant=w259) -> (data=→"Simulate\nconc":bool, error out=w256:errorcluster)
                }
                frame "calcon_save" {
                  n449 = Variant To Data(error in=w263, type=FALSE, Variant=w264) -> (data=→"calcon save to file":bool, error out=w261:errorcluster)
                }
                frame "mean_cal_status" {
                  n450 = Variant To Data(error in=w268, type=FALSE, Variant=w269) -> (data=→"Mean Cal\n(default = ON)":bool, error out=w266:errorcluster)
                }
              }
            }
            frame True {
            }
          }
          n451 = node-c288() -> ()  [unwired: 1 in, 1 out]
        }
        n452 = node-c288(w113) -> ()  [unwired: 1 out]
        n453 = Destroy Stream Endpoint(8:w118, 11:w117) -> (0:→"error out 4":errorcluster)
        n454 = Wait (ms)(milliseconds to wait=u32 1000) -> ()  [unwired: 1 out]
      }
      n455 = while {
        tunnel: w96 -> [w497]
        stop <- w498 stop-if-true
        # "UDP Broadcast loop"
        # "Broadcast UDP SO2 Data"
        n456 = node-c288() -> (w500:T4)  [unwired: 4 in]
        n457 = String To IP(1:"239.1.4.6" ("name")) -> (0:w502:u32)
        n458 = call-poly <vilib>:"UDP Multicast Open.vi"("time-to-live (1)"=u16 5, "port"=u16 10001) -> ("error out"=w510:errorcluster, "connection ID"=w511:refnum<k16>)  [unwired: 8 in]
        n459 = timed-loop {
          tunnel: w511 -> [w531]
          tunnel: w510 -> [w530]
          tunnel: [w517] -> w506
          shift-right: [w520] -> _
          shift-left: FALSE -> [w523]
          tunnel: [w515] -> w504
          tunnel: w502 -> [w519]
          tunnel: u16 50001 ("port or service name") -> [w518]
          timing: w500 -> [_]
          timing-out: [_] -> w499
          tunnel: [w513] -> w498
          tunnel: w497 -> [w512]
          stop <- w514 stop-if-true
          n460 = node-c288() -> ()  [unwired: 1 in, 1 out]
          n461 = local read "Flight Number"() -> (w526:string)
          n462 = Select(t=FALSE, s=w523, f=TRUE) -> (s? t:f=w520:bool)
          "UDP packet \nstatus" <- w520
          n463 = feedback-in #2(w526) -> ()
          n464 = feedback #2() -> (w525:string)  [unwired: 1 in]
          n465 = Not Equal?(x=w526, y=w525) -> (x != y?=w524:bool)
          n466 = flat-sequence {
            tunnel: w519 -> [w539]
            tunnel: w530 -> [w540]
            tunnel: w531 -> [w541]
            tunnel: [w541] -> w529
            tunnel: [w540] -> w528
            tunnel: [w539] -> w527
            tunnel: w524 -> [w538]
            tunnel: w518 -> [w551]
            tunnel: w529 -> [w550]
            tunnel: w528 -> [w549]
            tunnel: w527 -> [w548]
            tunnel: [w547] -> w517
            tunnel: [w546] -> w515
            tunnel: w512 -> [w545]
            frame #0 {
              n467 = feedback #3(u32 0) -> (w535:u32)
              n468 = case shown="True" w538 {
                tunnel: w535 -> [w542 _]
                tunnel: [w542 u32 0] -> w534
                frame False {
                }
                frame True {
                }
              }
              "UDP_Pack_num" <- w534
              n469 = Increment(x=w534) -> (x+1=w536:u32)
              n470 = feedback-in #3(w536) -> ()
            }
            frame #1 {
              n471 = Dequeue Element(queue=w545) -> (element=w544:string)  [unwired: 2 in, 3 out]
              n472 = UDP Write(address=w548, port or service name=w551, connection ID=w550, data in=w544, 8:w549) -> (error out=w546:errorcluster, 3:w547:refnum<k16>)  [unwired: 1 in]
            }
          }
          n473 = local read "stop"() -> (w513:bool)
          n474 = Unbundle(w515) -> ("status"=w516:bool)  [unwired: 2 out]
          n475 = node-c288() -> ()  [unwired: 1 in, 1 out]
          n476 = Compound Arithmetic op=OR(w516, w513) -> (w514:bool)
        }
        n477 = node-c288(w499) -> ()  [unwired: 1 out]
        n478 = UDP Close(connection ID=w506, 8:w504) -> (error out=→"UDP_Out_Error":errorcluster)  [unwired: 1 out]
        n479 = Wait (ms)(milliseconds to wait=u32 1000) -> ()  [unwired: 1 out]
      }
      n480 = while {
        tunnel: w94 -> [w456]
        tunnel: w95 -> [w455]
        stop <- w459 stop-if-true
        # "TCP Loop writing to SEPTIC Tank"
        n481 = TCP Open Connection(address="192.168.101.108", remote port or service name=u16 3502) -> (connection ID=w462:refnum<k5>, error out=w457:errorcluster)  [unwired: 3 in]
        n482 = case shown="No Error" w457 {
          selector: w457 -> [w467 w494]
          tunnel: w462 -> [w472 w495]
          tunnel: [w471 w495] -> w461
          tunnel: [w470 w494] -> w460
          tunnel: [w469 w493] -> w459
          tunnel: w455 -> [w466 _]
          tunnel: w456 -> [w465 _]
          frame No Error {
            n483 = node-c288() -> (w474:T4)  [unwired: 4 in]
            n484 = timed-loop {
              tunnel: w472 -> [w488]
              tunnel: w467 -> [w487]
              tunnel: [w486] -> w471
              tunnel: [w485] -> w470
              tunnel: [w475] -> w469
              shift-right: [w479] -> _
              shift-left: FALSE -> [w482]
              timing: w474 -> [_]
              timing-out: [_] -> w473
              tunnel: w466 -> [w478]
              tunnel: w465 -> [w477]
              stop <- w483 stop-if-true
              n485 = node-c288() -> ()  [unwired: 1 in, 1 out]
              n486 = Dequeue Element(queue=w478, error in (no error)=w477) -> (element=w476:string)  [unwired: 1 in, 3 out]
              n487 = Select(t=FALSE, s=w482, f=TRUE) -> (s? t:f=w479:bool)
              "TCP packet\nSend to SEPTIC" <- w479
              n488 = TCP Write(connection ID=w488, data in=w476, error in (no error)=w487) -> (connection ID out=w486:refnum<k5>, error out=w485:errorcluster)  [unwired: 1 in, 1 out]
              n489 = local read "stop"() -> (w475:bool)
              n490 = Unbundle(w485) -> ("status"=w484:bool)  [unwired: 2 out]
              n491 = node-c288() -> ()  [unwired: 1 in, 1 out]
              n492 = Compound Arithmetic op=OR(w484, w475) -> (w483:bool)
            }
            n493 = node-c288(w473) -> ()  [unwired: 1 out]
          }
          frame Error {
            n494 = local read "stop"() -> (w493:bool)
          }
        }
        n495 = TCP Close Connection(connection ID=w461, error in (no error)=w460) -> (error out=→"SEPTIC TCP Error Out":errorcluster)  [unwired: 1 in, 1 out]
        n496 = Wait (ms)(milliseconds to wait=u32 1000) -> ()  [unwired: 1 out]
      }
      n497 = while {
        tunnel: w100 -> [w556]
        tunnel: w99 -> [w555]
        stop <- w559 stop-if-true
        # "TCP Loop writing to FISH Tank"
        n498 = TCP Open Connection(address="192.168.101.110", remote port or service name=u16 3502) -> (connection ID=w562:refnum<k5>, error out=w557:errorcluster)  [unwired: 3 in]
        n499 = case shown="No Error" w557 {
          selector: w557 -> [w567 w594]
          tunnel: w562 -> [w572 w595]
          tunnel: [w571 w595] -> w561
          tunnel: [w570 w594] -> w560
          tunnel: [w569 w593] -> w559
          tunnel: w556 -> [w566 _]
          tunnel: w555 -> [w565 _]
          frame No Error {
            n500 = node-c288() -> (w574:T4)  [unwired: 4 in]
            n501 = timed-loop {
              tunnel: w572 -> [w588]
              tunnel: w567 -> [w587]
              tunnel: [w586] -> w571
              tunnel: [w585] -> w570
              tunnel: [w582] -> w569
              shift-right: [w578] -> _
              shift-left: FALSE -> [w581]
              timing: w574 -> [_]
              timing-out: [_] -> w573
              tunnel: w566 -> [w577]
              tunnel: w565 -> [w576]
              stop <- w583 stop-if-true
              n502 = node-c288() -> ()  [unwired: 1 in, 1 out]
              n503 = Dequeue Element(queue=w577, error in (no error)=w576) -> (element=w575:string)  [unwired: 1 in, 3 out]
              n504 = Select(t=FALSE, s=w581, f=TRUE) -> (s? t:f=w578:bool)
              "TCP packet\nSend to FISH" <- w578
              n505 = TCP Write(connection ID=w588, data in=w575, error in (no error)=w587) -> (connection ID out=w586:refnum<k5>, error out=w585:errorcluster)  [unwired: 1 in, 1 out]
              n506 = local read "stop"() -> (w582:bool)
              n507 = Unbundle(w585) -> ("status"=w584:bool)  [unwired: 2 out]
              n508 = node-c288() -> ()  [unwired: 1 in, 1 out]
              n509 = Compound Arithmetic op=OR(w584, w582) -> (w583:bool)
            }
            n510 = node-c288(w573) -> ()  [unwired: 1 out]
          }
          frame Error {
            n511 = local read "stop"() -> (w593:bool)
          }
        }
        n512 = TCP Close Connection(connection ID=w561, error in (no error)=w560) -> (error out=→"FISH TCP Error Out":errorcluster)  [unwired: 1 in, 1 out]
        n513 = Wait (ms)(milliseconds to wait=u32 1000) -> ()  [unwired: 1 out]
      }
    }
    frame Error {
    }
  }
  n514 = VISA Close(VISA resource name=w36, error in (no error)=w35) -> (error out=→"Serial Visa Error":errorcluster)
